vi "DDS_only.vi"() -> ()   [LabVIEW 2011]
doc: "I Description:\nThis example uses a script to manage the generation of a dynamic pattern at a specified clock rate.\n\nII Instructions for Running:\n1. Enter the digital channels on the hardware device to generate digital pattern in the Channel List control.\n2. Specify the clock rate for the generation in the Clock Rate control.\n3. Click the Stop button when you want to stop the generation\n\nIII Block Diagram Steps:\n1. Initialize for a generation session.\n2. Assign specified channels in Channel List for dynamic operation.\n3. Configure the Sample clock to use the onboard clock, and configure the clock rate.\n4. Set the generation mode to Scripted.\n5. Query the Data Width property to determine which Write function to use.\nNote: Different devices have different default values for the Data Width property. If you know the Data Width of your device, you may omit the property node and case structure.\n6. Write digital patterns to the onboard memory of the digital device.\n7. Write the script to the onboard memory.\n8. Initiate dynamic pattern generation.\n9. Wait until the Stop button is clicked or an error occurs, and exit the While loop. \n The niHSDIO Is Done VI is used in the while loop to check only for errors.\n10. Abort generation and close the session.\n\nIV I/O Connections Overview:\nMake connections from output terminals to match the channels specified by Channel List. In this example, the digital pattern is generated from the first 16 digital channels of the device."
uses:
  DDS drivers v3/DDS Settings.ctl
  DDS drivers v3/DDS RAM mode.ctl
  DDS drivers v3/DDS box device reference.ctl
  <vilib>/ni845x/ni845x.llb/ni845xControl.ctl
  ExperimentVariables/Variable_Settings.ctl
  <vilib>/Utility/error.llb/DialogType.ctl
  DDS drivers v3/AD9910 registers.ctl
  <vilib>/Utility/file.llb/Read From Spreadsheet File (string).vi
  ExperimentVariables/ExperimentVariables.lvclass
  DDS/DDS.lvclass
panel:
  in  "Quit Program":bool
  in  "Tab Control":enum32{"Experiment Variables", "DDS"}(tab)=enum."DDS"
  in  "Log":string="2012-07-23 09:53:31 Experiment ended\n\n2012-07-23 09:53:08 Experiment started\n\n2012-07-23 09:53:05 Experiment ended\n\n2012-07-23 09:52:53 Experiment started\n\n2012-07-23 09:52:48 Experiment ended\n\n2012-07-23 09:52:26 Experiment started\n\n2012-07-23 09:51:43 Experiment ended\n\n2012-07-23 09:46:17 Experiment started\n\n2012-07-23 09:44:29 Experiment ended\n\n2012-07-23 09:40:15 Experiment started\n\n2012-07-23 09:37:09 Experiment ended\n\n2012-07-23 09:32:48 Experiment started\n\n2012-07-23 09:32:41 Experiment ended\n\n2012-07-23 09:29:43 Experiment started\n\n2012-07-23 09:29:27 Experiment ended\n\n2012-07-23 09:26:51 Experiment started\n\n2012-07-23 09:26:22 Experiment ended\n\n2012-07-23 09:26:09 Experiment started\n\n2012-07-23 09:26:03 Experiment ended\n\n2012-07-23 09:25:53 Experiment started\n\n2012-07-23 09:25:46 Experiment ended\n\n2012-07-23 09:25:36 Experiment started\n\n2012-07-23 09:25:22 Experiment ended\n\n2012-07-23 09:25:08 Experiment started\n\n2012-07-23 09:24:58 Experiment ended\n\n2012-07-23 09:24:45 Experiment started\n\n2012-07-20 17:55:37 \n\nError cleared and continued by user\n\n2012-07-20 17:55:35 Warning 200010 occurred at DAQmx Stop Task.vi:4\r\n\r\nPossible reason(s):\n\r\nFinite acquisition or generation has been stopped before the requested number of samples were acquired or generated.\n\n2012-07-20 17:55:35 Experiment ended\n\n2012-07-20 17:54:26 Experiment started\n\n2012-07-20 17:53:50 Experiment ended\n\n2012-07-20 17:48:30 Experiment started\n\n2012-07-20 17:48:24 Experiment ended\n\n2012-07-20 17:43:48 Experiment started\n\n2012-07-20 17:43:47 Experiment ended\n\n2012-07-20 17:38:30 Experiment started\n\n2012-07-20 17:27:08 Experiment ended\n\n2012-07-20 17:26:09 Experiment started\n\n2012-07-20 17:25:58 \n\nError cleared and continued by user\n\n2012-07-20 17:25:57 Warning 200010 occurred at DAQmx Stop Task.vi:4\r\n\r\nPossible reason(s):\n\r\nFinite acquisition or generation has been stopped before the requested number of samples were acquired or generated.\n\n2012-07-20 17:25:57 Experiment ended\n\n2012-07-20 17:24:56 Experiment started\n\n2012-07-20 17:24:55 Experiment ended\n\n2012-07-20 17:19:07 Experiment started\n\n2012-07-20 16:57:52 Experiment ended\n\n2012-07-20 16:57:48 Experiment started\n\n2012-07-20 16:31:13 Experiment ended\n\n2012-07-20 16:28:51 Experiment started\n\n2012-07-20 16:26:58 \n\nError cleared and continued by user\n\n2012-07-20 16:26:56 Warning 200010 occurred at DAQmx Stop Task.vi:4\r\n\r\nPossible reason(s):\n\r\nFinite acquisition or generation has been stopped before the requested number of samples were acquired or generated.\n\n2012-07-20 16:26:56 Experiment ended\n\n2012-07-20 16:25:46 Experiment started\n\n2012-07-20 16:25:13 Experiment ended\n\n2012-07-20 16:25:06 Experiment started\n\n2012-07-20 16:20:49 Experiment ended\n\n2012-07-20 16:20:45 Warning:  The measurement ended due to the master timeout, before all output tasks were complete.  Consider increasing the timeout.\n\n2012-07-20 16:20:42 Warning:  The measurement ended due to the master timeout, before all output tasks were complete.  Consider increasing the timeout.\n\n2012-07-20 16:20:36 Warning:  The measurement ended due to the master timeout, before all output tasks were complete.  Consider increasing the timeout.\n\n2012-07-20 16:20:33 Warning:  The measurement ended due to the master timeout, before all output tasks were complete.  Consider increasing the timeout.\n\n2012-07-20 16:20:30 Warning:  The measurement ended due to the master timeout, before all output tasks were complete.  Consider increasing the timeout.\n\n2012-07-20 16:20:27 Warning:  The measurement ended due to the master timeout, before all output tasks were complete.  Consider increasing the timeout.\n\n2012-07-20 16:20:24 Warning:  The measurement ended due to the master timeout, before all output tasks were complete.  Consider increasing the timeout.\n\n2012-07-20 16:20:21 Warning:  The measurement ended due to the master timeout, before all output tasks were complete.  Consider increasing the timeout.\n\n2012-07-20 16:20:17 Warning:  The measurement ended due to the master timeout, before all output tasks were complete.  Consider increasing the timeout.\n\n2012-07-20 16:20:14 Warning:  The measurement ended due to the master timeout, before all output tasks were complete.  Consider increasing the timeout.\n\n2012-07-20 16:20:11 Warning:  The measurement ended due to the master timeout, before all output tasks were complete.  Consider increasing the timeout.\n\n2012-07-20 16:20:08 Warning:  The measurement ended due to the master timeout, before all output tasks were complete.  Consider increasing the timeout.\n\n2012-07-20 16:20:05 Warning:  The measurement ended due to the master timeout, before all output tasks were complete.  Consider increasing the timeout.\n\n2012-07-20 16:20:02 Warning:  The measurement ended due to the master timeout, before all output tasks were complete.  Consider increasing the timeout.\n\n2012-07-20 16:19:59 Warning:  The measurement ended due to the master timeout, before all output tasks were complete.  Consider increasing the timeout.\n\n2012-07-20 16:19:56 Warning:  The measurement ended due to the master timeout, before all output tasks were complete.  Consider increasing the timeout.\n\n2012-07-20 16:19:53 Warning:  The measurement ended due to the master timeout, before all output tasks were complete.  Consider increasing the timeout.\n\n2012-07-20 16:19:50 Warning:  The measurement ended due to the master timeout, before all output tasks were complete.  Consider increasing the timeout.\n\n2012-07-20 16:19:47 Warning:  The measurement ended due to the master timeout, before all output tasks were complete.  Consider increasing the timeout.\n\n2012-07-20 16:19:43 Warning:  The measurement ended due to the master timeout, before all output tasks were complete.  Consider increasing the timeout.\n\n2012-07-20 16:19:40 Warning:  The measurement ended due to the master timeout, before all output tasks were complete.  Consider increasing the timeout.\n\n2012-07-20 16:19:37 Warning:  The measurement ended due to the master timeout, before all output tasks were complete.  Consider increasing the timeout.\n\n2012-07-20 16:19:34 Warning:  The measurement ended due to the master timeout, before all output tasks were complete.  Consider increasing the timeout.\n\n2012-07-20 16:19:31 Warning:  The measurement ended due to the master timeout, before all output tasks were complete.  Consider increasing the timeout.\n\n2012-07-20 16:19:28 Warning:  The measurement ended due to the master timeout, before all output tasks were complete.  Consider increasing the timeout.\n\n2012-07-20 16:19:25 Warning:  The measurement ended due to the master timeout, before all output tasks were complete.  Consider increasing the timeout.\n\n2012-07-20 16:19:22 Warning:  The measurement ended due to the master timeout, before all output tasks were complete.  Consider increasing the timeout.\n\n2012-07-20 16:19:19 Warning:  The measurement ended due to the master timeout, before all output tasks were complete.  Consider increasing the timeout.\n\n2012-07-20 16:19:16 Experiment started\n\n2012-07-20 16:16:53 Experiment ended\n\n2012-07-20 16:16:51 Warning:  The measurement ended due to the master timeout, before all output tasks were complete.  Consider increasing the timeout.\n\n2012-07-20 16:16:48 Warning:  The measurement ended due to the master timeout, before all output tasks were complete.  Consider increasing the timeout.\n\n2012-07-20 16:16:45 Warning:  The measurement ended due to the master timeout, before all output tasks were complete.  Consider increasing the timeout.\n\n2012-07-20 16:16:42 Warning:  The measurement ended due to the master timeout, before all output tasks were complete.  Consider increasing the timeout.\n\n2012-07-20 16:16:39 Warning:  The measurement ended due to the master timeout, before all output tasks were complete.  Consider increasing the timeout.\n\n2012-07-20 16:16:36 Warning:  The measurement ended due to the master timeout, before all output tasks were complete.  Consider increasing the timeout.\n\n2012-07-20 16:16:33 Warning:  The measurement ended due to the master timeout, before all output tasks were complete.  Consider increasing the timeout.\n\n2012-07-20 16:16:29 Experiment started\n\n2012-07-20 16:15:09 Experiment ended\n\n2012-07-20 16:13:39 Warning:  The measurement ended due to the master timeout, before all output tasks were complete.  Consider increasing the timeout.\n\n2012-07-20 16:13:36 Warning:  The measurement ended due to the master timeout, before all output tasks were complete.  Consider increasing the timeout.\n\n2012-07-20 16:13:33 Warning:  The measurement ended due to the master timeout, before all output tasks were complete.  Consider increasing the timeout.\n\n2012-07-20 16:13:30 Warning:  The measurement ended due to the master timeout, before all output tasks were complete.  Consider increasing the timeout.\n\n2012-07-20 16:13:27 Warning:  The measurement ended due to the master timeout, before all output tasks were complete.  Consider increasing the timeout.\n\n2012-07-20 16:13:24 Warning:  The measurement ended due to the master timeout, before all output tasks were complete.  Consider increasing the timeout.\n\n2012-07-20 16:13:21 Warning:  The measurement ended due to the master timeout, before all output tasks were complete.  Consider increasing the timeout.\n\n2012-07-20 16:13:18 Warning:  The measurement ended due to the master timeout, before all output tasks were complete.  Consider increasing the timeout.\n\n2012-07-20 16:13:15 Warning:  The measurement ended due to the master timeout, before all output tasks were complete.  Consider increasing the timeout.\n\n2012-07-20 16:13:12 Warning:  The measurement ended due to the master timeout, before all output tasks were complete.  Consider increasing the timeout.\n\n2012-07-20 16:13:08 Warning:  The measurement ended due to the master timeout, before all output tasks were complete.  Consider increasing the timeout.\n\n2012-07-20 16:13:05 Warning:  The measurement ended due to the master timeout, before all output tasks were complete.  Consider increasing the timeout.\n\n2012-07-20 16:13:02 Warning:  The measurement ended due to the master timeout, before all output tasks were complete.  Consider increasing the timeout.\n\n2012-07-20 16:12:59 Warning:  The measurement ended due to the master timeout, before all output tasks were complete.  Consider increasing the timeout.\n\n2012-07-20 16:12:56 Warning:  The measurement ended due to the master timeout, before all output tasks were complete.  Consider increasing the timeout.\n\n2012-07-20 16:12:53 Warning:  The measurement ended due to the master timeout, before all output tasks were complete.  Consider increasing the timeout.\n\n2012-07-20 16:12:50 Warning:  The measurement ended due to the master timeout, before all output tasks were complete.  Consider increasing the timeout.\n\n2012-07-20 16:12:47 Warning:  The measurement ended due to the master timeout, before all output tasks were complete.  Consider increasing the timeout.\n\n2012-07-20 16:12:44 Warning:  The measurement ended due to the master timeout, before all output tasks were complete.  Consider increasing the timeout.\n\n2012-07-20 16:12:41 Warning:  The measurement ended due to the master timeout, before all output tasks were complete.  Consider increasing the timeout.\n\n2012-07-20 16:12:37 Warning:  The measurement ended due to the master timeout, before all output tasks were complete.  Consider increasing the timeout.\n\n2012-07-20 16:12:34 Warning:  The measurement ended due to the master timeout, before all output tasks were complete.  Consider increasing the timeout.\n\n2012-07-20 16:12:31 Warning:  The measurement ended due to the master timeout, before all output tasks were complete.  Consider increasing the timeout.\n\n2012-07-20 16:12:28 Warning:  The measurement ended due to the master timeout, before all output tasks were complete.  Consider increasing the timeout.\n\n2012-07-20 16:12:25 Warning:  The measurement ended due to the master timeout, before all output tasks were complete.  Consider increasing the timeout.\n\n2012-07-20 16:12:22 Warning:  The measurement ended due to the master timeout, before all output tasks were complete.  Consider increasing the timeout.\n\n2012-07-20 16:12:19 Warning:  The measurement ended due to the master timeout, before all output tasks were complete.  Consider increasing the timeout.\n\n2012-07-20 16:12:16 Warning:  The measurement ended due to the master timeout, before all output tasks were complete.  Consider increasing the timeout.\n\n2012-07-20 16:12:13 Warning:  The measurement ended due to the master timeout, before all output tasks were complete.  Consider increasing the timeout.\n\n2012-07-20 16:12:10 Warning:  The measurement ended due to the master timeout, before all output tasks were complete.  Consider increasing the timeout.\n\n2012-07-20 16:12:06 Warning:  The measurement ended due to the master timeout, before all output tasks were complete.  Consider increasing the timeout.\n\n2012-07-20 16:12:03 Warning:  The measurement ended due to the master timeout, before all output tasks were complete.  Consider increasing the timeout.\n\n2012-07-20 16:12:00 Warning:  The measurement ended due to the master timeout, before all output tasks were complete.  Consider increasing the timeout.\n\n2012-07-20 16:11:57 Warning:  The measurement ended due to the master timeout, before all output tasks were complete.  Consider increasing the timeout.\n\n2012-07-20 16:11:54 Warning:  The measurement ended due to the master timeout, before all output tasks were complete.  Consider increasing the timeout.\n\n2012-07-20 16:11:51 Warning:  The measurement ended due to the master timeout, before all output tasks were complete.  Consider increasing the timeout.\n\n2012-07-20 16:11:48 Warning:  The measurement ended due to the master timeout, before all output tasks were complete.  Consider increasing the timeout.\n\n2012-07-20 16:11:45 Warning:  The measurement ended due to the master timeout, before all output tasks were complete.  Consider increasing the timeout.\n\n2012-07-20 16:11:42 Warning:  The measurement ended due to the master timeout, before all output tasks were complete.  Consider increasing the timeout.\n\n2012-07-20 16:11:39 Warning:  The measurement ended due to the master timeout, before all output tasks were complete.  Consider increasing the timeout.\n\n2012-07-20 16:11:36 Warning:  The measurement ended due to the master timeout, before all output tasks were complete.  Consider increasing the timeout.\n\n2012-07-20 16:11:33 Warning:  The measurement ended due to the master timeout, before all output tasks were complete.  Consider increasing the timeout.\n\n2012-07-20 16:11:30 Warning:  The measurement ended due to the master timeout, before all output tasks were complete.  Consider increasing the timeout.\n\n2012-07-20 16:11:27 Warning:  The measurement ended due to the master timeout, before all output tasks were complete.  Consider increasing the timeout.\n\n2012-07-20 16:11:24 Warning:  The measurement ended due to the master timeout, before all output tasks were complete.  Consider increasing the timeout.\n\n2012-07-20 16:11:21 Warning:  The measurement ended due to the master timeout, before all output tasks were complete.  Consider increasing the timeout.\n\n2012-07-20 16:11:18 Warning:  The measurement ended due to the master timeout, before all output tasks were complete.  Consider increasing the timeout.\n\n2012-07-20 16:11:15 Warning:  The measurement ended due to the master timeout, before all output tasks were complete.  Consider increasing the timeout.\n\n2012-07-20 16:11:12 Warning:  The measurement ended due to the master timeout, before all output tasks were complete.  Consider increasing the timeout.\n\n2012-07-20 16:11:09 Warning:  The measurement ended due to the master timeout, before all output tasks were complete.  Consider increasing the timeout.\n\n2012-07-20 16:11:05 Warning:  The measurement ended due to the master timeout, before all output tasks were complete.  Consider increasing the timeout.\n\n2012-07-20 16:11:02 Warning:  The measurement ended due to the master timeout, before all output tasks were complete.  Consider increasing the timeout.\n\n2012-07-20 16:10:59 Warning:  The measurement ended due to the master timeout, before all output tasks were complete.  Consider increasing the timeout.\n\n2012-07-20 16:10:56 Warning:  The measurement ended due to the master timeout, before all output tasks were complete.  Consider increasing the timeout.\n\n2012-07-20 16:10:53 Warning:  The measurement ended due to the master timeout, before all output tasks were complete.  Consider increasing the timeout.\n\n2012-07-20 16:10:50 Warning:  The measurement ended due to the master timeout, before all output tasks were complete.  Consider increasing the timeout.\n\n2012-07-20 16:10:47 Warning:  The measurement ended due to the master timeout, before all output tasks were complete.  Consider increasing the timeout.\n\n2012-07-20 16:10:44 Warning:  The measurement ended due to the master timeout, before all output tasks were complete.  Consider increasing the timeout.\n\n2012-07-20 16:10:41 Warning:  The measurement ended due to the master timeout, before all output tasks were complete.  Consider increasing the timeout.\n\n2012-07-20 16:10:38 Warning:  The measurement ended due to the master timeout, before all output tasks were complete.  Consider increasing the timeout.\n\n2012-07-20 16:10:34 Warning:  The measurement ended due to the master timeout, before all output tasks were complete.  Consider increasing the timeout.\n\n2012-07-20 16:10:31 Warning:  The measurement ended due to the master timeout, before all output tasks were complete.  Consider increasing the timeout.\n\n2012-07-20 16:10:28 Warning:  The measurement ended due to the master timeout, before all output tasks were complete.  Consider increasing the timeout.\n\n2012-07-20 16:10:25 Warning:  The measurement ended due to the master timeout, before all output tasks were complete.  Consider increasing the timeout.\n\n2012-07-20 16:10:22 Warning:  The measurement ended due to the master timeout, before all output tasks were complete.  Consider increasing the timeout.\n\n2012-07-20 16:10:19 Warning:  The measurement ended due to the master timeout, before all output tasks were complete.  Consider increasing the timeout.\n\n2012-07-20 16:10:16 Warning:  The measurement ended due to the master timeout, before all output tasks were complete.  Consider increasing the timeout.\n\n2012-07-20 16:10:13 Warning:  The measurement ended due to the master timeout, before all output tasks were complete.  Consider increasing the timeout.\n\n2012-07-20 16:10:10 Warning:  The measurement ended due to the master timeout, before all output tasks were complete.  Consider increasing the timeout.\n\n2012-07-20 16:10:07 Warning:  The measurement ended due to the master timeout, before all output tasks were complete.  Consider increasing the timeout.\n\n2012-07-20 16:10:03 Warning:  The measurement ended due to the master timeout, before all output tasks were complete.  Consider increasing the timeout.\n\n2012-07-20 16:10:00 Warning:  The measurement ended due to the master timeout, before all output tasks were complete.  Consider increasing the timeout.\n\n2012-07-20 16:09:57 Warning:  The measurement ended due to the master timeout, before all output tasks were complete.  Consider increasing the timeout.\n\n2012-07-20 16:09:54 Warning:  The measurement ended due to the master timeout, before all output tasks were complete.  Consider increasing the timeout.\n\n2012-07-20 16:09:51 Warning:  The measurement ended due to the master timeout, before all output tasks were complete.  Consider increasing the timeout.\n\n2012-07-20 16:09:48 Warning:  The measurement ended due to the master timeout, before all output tasks were complete.  Consider increasing the timeout.\n\n2012-07-20 16:09:45 Warning:  The measurement ended due to the master timeout, before all output tasks were complete.  Consider increasing the timeout.\n\n2012-07-20 16:09:42 Warning:  The measurement ended due to the master timeout, before all output tasks were complete.  Consider increasing the timeout.\n\n2012-07-20 16:09:39 Warning:  The measurement ended due to the master timeout, before all output tasks were complete.  Consider increasing the timeout.\n\n2012-07-20 16:09:36 Warning:  The measurement ended due to the master timeout, before all output tasks were complete.  Consider increasing the timeout.\n\n2012-07-20 16:09:33 Warning:  The measurement ended due to the master timeout, before all output tasks were complete.  Consider increasing the timeout.\n\n2012-07-20 16:09:30 Warning:  The measurement ended due to the master timeout, before all output tasks were complete.  Consider increasing the timeout.\n\n2012-07-20 16:09:27 Warning:  The measurement ended due to the master timeout, before all output tasks were complete.  Consider increasing the timeout.\n\n2012-07-20 16:09:24 Warning:  The measurement ended due to the master timeout, before all output tasks were complete.  Consider increasing the timeout.\n\n2012-07-20 16:09:21 Warning:  The measurement ended due to the master timeout, before all output tasks were complete.  Consider increasing the timeout.\n\n2012-07-20 16:09:18 Warning:  The measurement ended due to the master timeout, before all output tasks were complete.  Consider increasing the timeout.\n\n2012-07-20 16:09:15 Warning:  The measurement ended due to the master timeout, before all output tasks were complete.  Consider increasing the timeout.\n\n2012-07-20 16:09:12 Warning:  The measurement ended due to the master timeout, before all output tasks were complete.  Consider increasing the timeout.\n\n2012-07-20 16:09:09 Warning:  The measurement ended due to the master timeout, before all output tasks were complete.  Consider increasing the timeout.\n\n2012-07-20 16:09:06 Warning:  The measurement ended due to the master timeout, before all output tasks were complete.  Consider increasing the timeout.\n\n2012-07-20 16:09:02 Warning:  The measurement ended due to the master timeout, before all output tasks were complete.  Consider increasing the timeout.\n\n2012-07-20 16:08:59 Warning:  The measurement ended due to the master timeout, before all output tasks were complete.  Consider increasing the timeout.\n\n2012-07-20 16:08:56 Warning:  The measurement ended due to the master timeout, before all output tasks were complete.  Consider increasing the timeout.\n\n2012-07-20 16:08:53 Warning:  The measurement ended due to the master timeout, before all output tasks were complete.  Consider increasing the timeout.\n\n2012-07-20 16:08:50 Warning:  The measurement ended due to the master timeout, before all output tasks were complete.  Consider increasing the timeout.\n\n2012-07-20 16:08:47 Warning:  The measurement ended due to the master timeout, before all output tasks were complete.  Consider increasing the timeout.\n\n2012-07-20 16:08:44 Warning:  The measurement ended due to the master timeout, before all output tasks were complete.  Consider increasing the timeout.\n\n2012-07-20 16:08:38 Warning:  The measurement ended due to the master timeout, before all output tasks were complete.  Consider increasing the timeout.\n\n2012-07-20 16:08:35 Warning:  The measurement ended due to the master timeout, before all output tasks were complete.  Consider increasing the timeout.\n\n2012-07-20 16:08:31 Warning:  The measurement ended due to the master timeout, before all output tasks were complete.  Consider increasing the timeout.\n\n2012-07-20 16:08:28 Warning:  The measurement ended due to the master timeout, before all output tasks were complete.  Consider increasing the timeout.\n\n2012-07-20 16:08:25 Warning:  The measurement ended due to the master timeout, before all output tasks were complete.  Consider increasing the timeout.\n\n2012-07-20 16:08:22 Warning:  The measurement ended due to the master timeout, before all output tasks were complete.  Consider increasing the timeout.\n\n2012-07-20 16:08:19 Warning:  The measurement ended due to the master timeout, before all output tasks were complete.  Consider increasing the timeout.\n\n2012-07-20 16:08:16 Warning:  The measurement ended due to the master timeout, before all output tasks were complete.  Consider increasing the timeout.\n\n2012-07-20 16:08:13 Warning:  The measurement ended due to the master timeout, before all output tasks were complete.  Consider increasing the timeout.\n\n2012-07-20 16:08:10 Warning:  The measurement ended due to the master timeout, before all output tasks were complete.  Consider increasing the timeout.\n\n2012-07-20 16:08:07 Warning:  The measurement ended due to the master timeout, before all output tasks were complete.  Consider increasing the timeout.\n\n2012-07-20 16:08:04 Warning:  The measurement ended due to the master timeout, before all output tasks were complete.  Consider increasing the timeout.\n\n2012-07-20 16:08:00 Experiment started\n\n2012-07-20 16:07:21 \n\nHalted by user.\n\n2012-07-20 16:07:18 Error -50103 occurred at Analog_Output.lvclass:update.vi\r\n\r\nPossible reason(s):\n\r\nNI Platform Services:  The specified resource is reserved. The operation could not be completed as specified.\r\n\nTask Name: _unnamedTask<185>\n\n2012-07-20 16:07:18 Experiment ended\n\n2012-07-20 16:07:16 Experiment started\n\n2012-07-20 16:07:16 \n\nError cleared and continued by user\n\n2012-07-20 16:07:14 Error 100 occurred at DDS Com Error\r\n\r\nPossible reason(s):\n\r\nLabVIEW:  File contains erroneous data. This normally is a user data file.\n\n2012-07-20 16:07:14 Experiment ended\n\n2012-07-20 16:07:12 Experiment started\n\n2012-07-20 16:06:57 \n\nHalted by user.\n\n2012-07-20 16:06:46 Error 100 occurred at DDS Com Error\r\n\r\nPossible reason(s):\n\r\nLabVIEW:  File contains erroneous data. This normally is a user data file.\n\n2012-07-20 16:06:46 Experiment ended\n\n2012-07-20 16:06:38 Experiment started\n\n2012-07-20 16:06:13 \n\nError cleared and continued by user\n\n2012-07-20 16:06:10 Error 100 occurred at DDS Com Error\r\n\r\nPossible reason(s):\n\r\nLabVIEW:  File contains erroneous data. This normally is a user data file.\n\n2012-07-20 16:06:10 Experiment ended\n\n2012-07-20 16:06:06 Experiment started\n\n2012-07-20 16:05:54 \n\nError cleared and continued by user\n\n2012-07-20 16:05:52 Error 100 occurred at DDS Com Error\r\n\r\nPossible reason(s):\n\r\nLabVIEW:  File contains erroneous data. This normally is a user data file.\n\n2012-07-20 16:05:52 Experiment ended\n\n2012-07-20 16:05:49 Experiment started\n\n2012-07-20 16:05:16 Experiment ended\n\n2012-07-20 16:04:44 Warning:  The measurement ended due to the master timeout, before all output tasks were complete.  Consider increasing the timeout.\n\n2012-07-20 16:04:41 Warning:  The measurement ended due to the master timeout, before all output tasks were complete.  Consider increasing the timeout.\n\n2012-07-20 16:04:38 Warning:  The measurement ended due to the master timeout, before all output tasks were complete.  Consider increasing the timeout.\n\n2012-07-20 16:04:35 Warning:  The measurement ended due to the master timeout, before all output tasks were complete.  Consider increasing the timeout.\n\n2012-07-20 16:04:31 Warning:  The measurement ended due to the master timeout, before all output tasks were complete.  Consider increasing the timeout.\n\n2012-07-20 16:04:28 Warning:  The measurement ended due to the master timeout, before all output tasks were complete.  Consider increasing the timeout.\n\n2012-07-20 16:04:25 Warning:  The measurement ended due to the master timeout, before all output tasks were complete.  Consider increasing the timeout.\n\n2012-07-20 16:04:22 Warning:  The measurement ended due to the master timeout, before all output tasks were complete.  Consider increasing the timeout.\n\n2012-07-20 16:04:19 Warning:  The measurement ended due to the master timeout, before all output tasks were complete.  Consider increasing the timeout.\n\n2012-07-20 16:04:16 Warning:  The measurement ended due to the master timeout, before all output tasks were complete.  Consider increasing the timeout.\n\n2012-07-20 16:04:13 Warning:  The measurement ended due to the master timeout, before all output tasks were complete.  Consider increasing the timeout.\n\n2012-07-20 16:04:10 Warning:  The measurement ended due to the master timeout, before all output tasks were complete.  Consider increasing the timeout.\n\n2012-07-20 16:04:07 Warning:  The measurement ended due to the master timeout, before all output tasks were complete.  Consider increasing the timeout.\n\n2012-07-20 16:04:04 Warning:  The measurement ended due to the master timeout, before all output tasks were complete.  Consider increasing the timeout.\n\n2012-07-20 16:04:01 Warning:  The measurement ended due to the master timeout, before all output tasks were complete.  Consider increasing the timeout.\n\n2012-07-20 16:03:58 Warning:  The measurement ended due to the master timeout, before all output tasks were complete.  Consider increasing the timeout.\n\n2012-07-20 16:03:55 Warning:  The measurement ended due to the master timeout, before all output tasks were complete.  Consider increasing the timeout.\n\n2012-07-20 16:03:51 Warning:  The measurement ended due to the master timeout, before all output tasks were complete.  Consider increasing the timeout.\n\n2012-07-20 16:03:48 Warning:  The measurement ended due to the master timeout, before all output tasks were complete.  Consider increasing the timeout.\n\n2012-07-20 16:03:45 Warning:  The measurement ended due to the master timeout, before all output tasks were complete.  Consider increasing the timeout.\n\n2012-07-20 16:03:42 Warning:  The measurement ended due to the master timeout, before all output tasks were complete.  Consider increasing the timeout.\n\n2012-07-20 16:03:39 Warning:  The measurement ended due to the master timeout, before all output tasks were complete.  Consider increasing the timeout.\n\n2012-07-20 16:03:36 Warning:  The measurement ended due to the master timeout, before all output tasks were complete.  Consider increasing the timeout.\n\n2012-07-20 16:03:33 Warning:  The measurement ended due to the master timeout, before all output tasks were complete.  Consider increasing the timeout.\n\n2012-07-20 16:03:30 Warning:  The measurement ended due to the master timeout, before all output tasks were complete.  Consider increasing the timeout.\n\n2012-07-20 16:03:27 Warning:  The measurement ended due to the master timeout, before all output tasks were complete.  Consider increasing the timeout.\n\n2012-07-20 16:03:24 Warning:  The measurement ended due to the master timeout, before all output tasks were complete.  Consider increasing the timeout.\n\n2012-07-20 16:03:21 Warning:  The measurement ended due to the master timeout, before all output tasks were complete.  Consider increasing the timeout.\n\n2012-07-20 16:03:18 Warning:  The measurement ended due to the master timeout, before all output tasks were complete.  Consider increasing the timeout.\n\n2012-07-20 16:03:15 Warning:  The measurement ended due to the master timeout, before all output tasks were complete.  Consider increasing the timeout.\n\n2012-07-20 16:03:12 Warning:  The measurement ended due to the master timeout, before all output tasks were complete.  Consider increasing the timeout.\n\n2012-07-20 16:03:09 Warning:  The measurement ended due to the master timeout, before all output tasks were complete.  Consider increasing the timeout.\n\n2012-07-20 16:03:05 Warning:  The measurement ended due to the master timeout, before all output tasks were complete.  Consider increasing the timeout.\n\n2012-07-20 16:03:02 Warning:  The measurement ended due to the master timeout, before all output tasks were complete.  Consider increasing the timeout.\n\n2012-07-20 16:02:59 Warning:  The measurement ended due to the master timeout, before all output tasks were complete.  Consider increasing the timeout.\n\n2012-07-20 16:02:56 Warning:  The measurement ended due to the master timeout, before all output tasks were complete.  Consider increasing the timeout.\n\n2012-07-20 16:02:53 Warning:  The measurement ended due to the master timeout, before all output tasks were complete.  Consider increasing the timeout.\n\n2012-07-20 16:02:50 Warning:  The measurement ended due to the master timeout, before all output tasks were complete.  Consider increasing the timeout.\n\n2012-07-20 16:02:47 Warning:  The measurement ended due to the master timeout, before all output tasks were complete.  Consider increasing the timeout.\n\n2012-07-20 16:02:44 Warning:  The measurement ended due to the master timeout, before all output tasks were complete.  Consider increasing the timeout.\n\n2012-07-20 16:02:41 Warning:  The measurement ended due to the master timeout, before all output tasks were complete.  Consider increasing the timeout.\n\n2012-07-20 16:02:38 Warning:  The measurement ended due to the master timeout, before all output tasks were complete.  Consider increasing the timeout.\n\n2012-07-20 16:02:35 Warning:  The measurement ended due to the master timeout, before all output tasks were complete.  Consider increasing the timeout.\n\n2012-07-20 16:02:32 Warning:  The measurement ended due to the master timeout, before all output tasks were complete.  Consider increasing the timeout.\n\n2012-07-20 16:02:28 Warning:  The measurement ended due to the master timeout, before all output tasks were complete.  Consider increasing the timeout.\n\n2012-07-20 16:02:25 Warning:  The measurement ended due to the master timeout, before all output tasks were complete.  Consider increasing the timeout.\n\n2012-07-20 16:02:19 Warning:  The measurement ended due to the master timeout, before all output tasks were complete.  Consider increasing the timeout.\n\n2012-07-20 16:02:16 Warning:  The measurement ended due to the master timeout, before all output tasks were complete.  Consider increasing the timeout.\n\n2012-07-20 16:02:13 Warning:  The measurement ended due to the master timeout, before all output tasks were complete.  Consider increasing the timeout.\n\n2012-07-20 16:02:10 Warning:  The measurement ended due to the master timeout, before all output tasks were complete.  Consider increasing the timeout.\n\n2012-07-20 16:02:07 Warning:  The measurement ended due to the master timeout, before all output tasks were complete.  Consider increasing the timeout.\n\n2012-07-20 16:02:04 Warning:  The measurement ended due to the master timeout, before all output tasks were complete.  Consider increasing the timeout.\n\n2012-07-20 16:02:01 Warning:  The measurement ended due to the master timeout, before all output tasks were complete.  Consider increasing the timeout.\n\n2012-07-20 16:01:57 Warning:  The measurement ended due to the master timeout, before all output tasks were complete.  Consider increasing the timeout.\n\n2012-07-20 16:01:54 Warning:  The measurement ended due to the master timeout, before all output tasks were complete.  Consider increasing the timeout.\n\n2012-07-20 16:01:51 Warning:  The measurement ended due to the master timeout, before all output tasks were complete.  Consider increasing the timeout.\n\n2012-07-20 16:01:48 Warning:  The measurement ended due to the master timeout, before all output tasks were complete.  Consider increasing the timeout.\n\n2012-07-20 16:01:45 Warning:  The measurement ended due to the master timeout, before all output tasks were complete.  Consider increasing the timeout.\n\n2012-07-20 16:01:42 Warning:  The measurement ended due to the master timeout, before all output tasks were complete.  Consider increasing the timeout.\n\n2012-07-20 16:01:39 Warning:  The measurement ended due to the master timeout, before all output tasks were complete.  Consider increasing the timeout.\n\n2012-07-20 16:01:36 Warning:  The measurement ended due to the master timeout, before all output tasks were complete.  Consider increasing the timeout.\n\n2012-07-20 16:01:33 Warning:  The measurement ended due to the master timeout, before all output tasks were complete.  Consider increasing the timeout.\n\n2012-07-20 16:01:30 Warning:  The measurement ended due to the master timeout, before all output tasks were complete.  Consider increasing the timeout.\n\n2012-07-20 16:01:23 Warning:  The measurement ended due to the master timeout, before all output tasks were complete.  Consider increasing the timeout.\n\n2012-07-20 16:01:20 Warning:  The measurement ended due to the master timeout, before all output tasks were complete.  Consider increasing the timeout.\n\n2012-07-20 16:01:17 Warning:  The measurement ended due to the master timeout, before all output tasks were complete.  Consider increasing the timeout.\n\n2012-07-20 16:01:14 Warning:  The measurement ended due to the master timeout, before all output tasks were complete.  Consider increasing the timeout.\n\n2012-07-20 16:01:11 Warning:  The measurement ended due to the master timeout, before all output tasks were complete.  Consider increasing the timeout.\n\n2012-07-20 16:01:08 Warning:  The measurement ended due to the master timeout, before all output tasks were complete.  Consider increasing the timeout.\n\n2012-07-20 16:01:05 Warning:  The measurement ended due to the master timeout, before all output tasks were complete.  Consider increasing the timeout.\n\n2012-07-20 16:01:02 Warning:  The measurement ended due to the master timeout, before all output tasks were complete.  Consider increasing the timeout.\n\n2012-07-20 16:00:59 Warning:  The measurement ended due to the master timeout, before all output tasks were complete.  Consider increasing the timeout.\n\n2012-07-20 16:00:55 Warning:  The measurement ended due to the master timeout, before all output tasks were complete.  Consider increasing the timeout.\n\n2012-07-20 16:00:52 Warning:  The measurement ended due to the master timeout, before all output tasks were complete.  Consider increasing the timeout.\n\n2012-07-20 16:00:49 Warning:  The measurement ended due to the master timeout, before all output tasks were complete.  Consider increasing the timeout.\n\n2012-07-20 16:00:46 Warning:  The measurement ended due to the master timeout, before all output tasks were complete.  Consider increasing the timeout.\n\n2012-07-20 16:00:43 Warning:  The measurement ended due to the master timeout, before all output tasks were complete.  Consider increasing the timeout.\n\n2012-07-20 16:00:40 Warning:  The measurement ended due to the master timeout, before all output tasks were complete.  Consider increasing the timeout.\n\n2012-07-20 16:00:37 Warning:  The measurement ended due to the master timeout, before all output tasks were complete.  Consider increasing the timeout.\n\n2012-07-20 16:00:34 Warning:  The measurement ended due to the master timeout, before all output tasks were complete.  Consider increasing the timeout.\n\n2012-07-20 16:00:31 Warning:  The measurement ended due to the master timeout, before all output tasks were complete.  Consider increasing the timeout.\n\n2012-07-20 16:00:28 Warning:  The measurement ended due to the master timeout, before all output tasks were complete.  Consider increasing the timeout.\n\n2012-07-20 16:00:25 Warning:  The measurement ended due to the master timeout, before all output tasks were complete.  Consider increasing the timeout.\n\n2012-07-20 16:00:21 Warning:  The measurement ended due to the master timeout, before all output tasks were complete.  Consider increasing the timeout.\n\n2012-07-20 16:00:18 Warning:  The measurement ended due to the master timeout, before all output tasks were complete.  Consider increasing the timeout.\n\n2012-07-20 16:00:15 Warning:  The measurement ended due to the master timeout, before all output tasks were complete.  Consider increasing the timeout.\n\n2012-07-20 16:00:12 Warning:  The measurement ended due to the master timeout, before all output tasks were complete.  Consider increasing the timeout.\n\n2012-07-20 16:00:09 Warning:  The measurement ended due to the master timeout, before all output tasks were complete.  Consider increasing the timeout.\n\n2012-07-20 16:00:06 Warning:  The measurement ended due to the master timeout, before all output tasks were complete.  Consider increasing the timeout.\n\n2012-07-20 16:00:03 Warning:  The measurement ended due to the master timeout, before all output tasks were complete.  Consider increasing the timeout.\n\n2012-07-20 16:00:00 Warning:  The measurement ended due to the master timeout, before all output tasks were complete.  Consider increasing the timeout.\n\n2012-07-20 15:59:57 Warning:  The measurement ended due to the master timeout, before all output tasks were complete.  Consider increasing the timeout.\n\n2012-07-20 15:59:54 Experiment started\n\n2012-07-20 15:59:36 \n\nError cleared and continued by user\n\n2012-07-20 15:59:35 Warning 200010 occurred at DAQmx Stop Task.vi:4\r\n\r\nPossible reason(s):\n\r\nFinite acquisition or generation has been stopped before the requested number of samples were acquired or generated.\n\n2012-07-20 15:59:35 Experiment ended\n\n2012-07-20 15:57:39 Experiment started\n\n2012-07-20 15:52:08 \n\nError cleared and continued by user\n\n2012-07-20 15:52:06 Warning 200010 occurred at DAQmx Stop Task.vi:4\r\n\r\nPossible reason(s):\n\r\nFinite acquisition or generation has been stopped before the requested number of samples were acquired or generated.\n\n2012-07-20 15:52:06 Experiment ended\n\n2012-07-20 15:52:03 Warning:  The measurement ended due to the master timeout, before all output tasks were complete.  Consider increasing the timeout.\n\n2012-07-20 15:52:00 Warning:  The measurement ended due to the master timeout, before all output tasks were complete.  Consider increasing the timeout.\n\n2012-07-20 15:51:57 Warning:  The measurement ended due to the master timeout, before all output tasks were complete.  Consider increasing the timeout.\n\n2012-07-20 15:51:54 Warning:  The measurement ended due to the master timeout, before all output tasks were complete.  Consider increasing the timeout.\n\n2012-07-20 15:51:51 Warning:  The measurement ended due to the master timeout, before all output tasks were complete.  Consider increasing the timeout.\n\n2012-07-20 15:51:48 Warning:  The measurement ended due to the master timeout, before all output tasks were complete.  Consider increasing the timeout.\n\n2012-07-20 15:51:45 Warning:  The measurement ended due to the master timeout, before all output tasks were complete.  Consider increasing the timeout.\n\n2012-07-20 15:51:42 Warning:  The measurement ended due to the master timeout, before all output tasks were complete.  Consider increasing the timeout.\n\n2012-07-20 15:51:39 Warning:  The measurement ended due to the master timeout, before all output tasks were complete.  Consider increasing the timeout.\n\n2012-07-20 15:51:36 Warning:  The measurement ended due to the master timeout, before all output tasks were complete.  Consider increasing the timeout.\n\n2012-07-20 15:51:33 Warning:  The measurement ended due to the master timeout, before all output tasks were complete.  Consider increasing the timeout.\n\n2012-07-20 15:51:30 Warning:  The measurement ended due to the master timeout, before all output tasks were complete.  Consider increasing the timeout.\n\n2012-07-20 15:51:27 Warning:  The measurement ended due to the master timeout, before all output tasks were complete.  Consider increasing the timeout.\n\n2012-07-20 15:51:24 Warning:  The measurement ended due to the master timeout, before all output tasks were complete.  Consider increasing the timeout.\n\n2012-07-20 15:51:21 Warning:  The measurement ended due to the master timeout, before all output tasks were complete.  Consider increasing the timeout.\n\n2012-07-20 15:51:18 Warning:  The measurement ended due to the master timeout, before all output tasks were complete.  Consider increasing the timeout.\n\n2012-07-20 15:51:15 Warning:  The measurement ended due to the master timeout, before all output tasks were complete.  Consider increasing the timeout.\n\n2012-07-20 15:51:12 Warning:  The measurement ended due to the master timeout, before all output tasks were complete.  Consider increasing the timeout.\n\n2012-07-20 15:51:09 Warning:  The measurement ended due to the master timeout, before all output tasks were complete.  Consider increasing the timeout.\n\n2012-07-20 15:51:02 Warning:  The measurement ended due to the master timeout, before all output tasks were complete.  Consider increasing the timeout.\n\n2012-07-20 15:50:59 Warning:  The measurement ended due to the master timeout, before all output tasks were complete.  Consider increasing the timeout.\n\n2012-07-20 15:50:56 Warning:  The measurement ended due to the master timeout, before all output tasks were complete.  Consider increasing the timeout.\n\n2012-07-20 15:50:53 Warning:  The measurement ended due to the master timeout, before all output tasks were complete.  Consider increasing the timeout.\n\n2012-07-20 15:50:50 Warning:  The measurement ended due to the master timeout, before all output tasks were complete.  Consider increasing the timeout.\n\n2012-07-20 15:50:44 Warning:  The measurement ended due to the master timeout, before all output tasks were complete.  Consider increasing the timeout.\n\n2012-07-20 15:50:41 Warning:  The measurement ended due to the master timeout, before all output tasks were complete.  Consider increasing the timeout.\n\n2012-07-20 15:50:38 Warning:  The measurement ended due to the master timeout, before all output tasks were complete.  Consider increasing the timeout.\n\n2012-07-20 15:50:35 Warning:  The measurement ended due to the master timeout, before all output tasks were complete.  Consider increasing the timeout.\n\n2012-07-20 15:50:32 Warning:  The measurement ended due to the master timeout, before all output tasks were complete.  Consider increasing the timeout.\n\n2012-07-20 15:50:29 Warning:  The measurement ended due to the master timeout, before all output tasks were complete.  Consider increasing the timeout.\n\n2012-07-20 15:50:26 Warning:  The measurement ended due to the master timeout, before all output tasks were complete.  Consider increasing the timeout.\n\n2012-07-20 15:50:23 Warning:  The measurement ended due to the master timeout, before all output tasks were complete.  Consider increasing the timeout.\n\n2012-07-20 15:50:20 Warning:  The measurement ended due to the master timeout, before all output tasks were complete.  Consider increasing the timeout.\n\n2012-07-20 15:50:17 Warning:  The measurement ended due to the master timeout, before all output tasks were complete.  Consider increasing the timeout.\n\n2012-07-20 15:50:14 Warning:  The measurement ended due to the master timeout, before all output tasks were complete.  Consider increasing the timeout.\n\n2012-07-20 15:50:11 Warning:  The measurement ended due to the master timeout, before all output tasks were complete.  Consider increasing the timeout.\n\n2012-07-20 15:50:08 Warning:  The measurement ended due to the master timeout, before all output tasks were complete.  Consider increasing the timeout.\n\n2012-07-20 15:50:05 Warning:  The measurement ended due to the master timeout, before all output tasks were complete.  Consider increasing the timeout.\n\n2012-07-20 15:50:02 Warning:  The measurement ended due to the master timeout, before all output tasks were complete.  Consider increasing the timeout.\n\n2012-07-20 15:49:56 Warning:  The measurement ended due to the master timeout, before all output tasks were complete.  Consider increasing the timeout.\n\n2012-07-20 15:49:53 Warning:  The measurement ended due to the master timeout, before all output tasks were complete.  Consider increasing the timeout.\n\n2012-07-20 15:49:50 Warning:  The measurement ended due to the master timeout, before all output tasks were complete.  Consider increasing the timeout.\n\n2012-07-20 15:49:47 Warning:  The measurement ended due to the master timeout, before all output tasks were complete.  Consider increasing the timeout.\n\n2012-07-20 15:49:44 Warning:  The measurement ended due to the master timeout, before all output tasks were complete.  Consider increasing the timeout.\n\n2012-07-20 15:49:41 Warning:  The measurement ended due to the master timeout, before all output tasks were complete.  Consider increasing the timeout.\n\n2012-07-20 15:49:38 Warning:  The measurement ended due to the master timeout, before all output tasks were complete.  Consider increasing the timeout.\n\n2012-07-20 15:49:35 Warning:  The measurement ended due to the master timeout, before all output tasks were complete.  Consider increasing the timeout.\n\n2012-07-20 15:49:32 Warning:  The measurement ended due to the master timeout, before all output tasks were complete.  Consider increasing the timeout.\n\n2012-07-20 15:49:29 Warning:  The measurement ended due to the master timeout, before all output tasks were complete.  Consider increasing the timeout.\n\n2012-07-20 15:49:26 Warning:  The measurement ended due to the master timeout, before all output tasks were complete.  Consider increasing the timeout.\n\n2012-07-20 15:49:23 Warning:  The measurement ended due to the master timeout, before all output tasks were complete.  Consider increasing the timeout.\n\n2012-07-20 15:33:14 Warning:  The measurement ended due to the master timeout, before all output tasks were complete.  Consider increasing the timeout.\n\n2012-07-20 15:33:08 Warning:  The measurement ended due to the master timeout, before all output tasks were complete.  Consider increasing the timeout.\n\n2012-07-20 15:33:05 Warning:  The measurement ended due to the master timeout, before all output tasks were complete.  Consider increasing the timeout.\n\n2012-07-20 15:33:02 Warning:  The measurement ended due to the master timeout, before all output tasks were complete.  Consider increasing the timeout.\n\n2012-07-20 15:32:59 Warning:  The measurement ended due to the master timeout, before all output tasks were complete.  Consider increasing the timeout.\n\n2012-07-20 15:32:56 Warning:  The measurement ended due to the master timeout, before all output tasks were complete.  Consider increasing the timeout.\n\n2012-07-20 15:32:53 Warning:  The measurement ended due to the master timeout, before all output tasks were complete.  Consider increasing the timeout.\n\n2012-07-20 15:32:50 Warning:  The measurement ended due to the master timeout, before all output tasks were complete.  Consider increasing the timeout.\n\n2012-07-20 15:32:47 Warning:  The measurement ended due to the master timeout, before all output tasks were complete.  Consider increasing the timeout.\n\n2012-07-20 15:32:44 Warning:  The measurement ended due to the master timeout, before all output tasks were complete.  Consider increasing the timeout.\n\n2012-07-20 15:32:41 Warning:  The measurement ended due to the master timeout, before all output tasks were complete.  Consider increasing the timeout.\n\n2012-07-20 15:32:38 Warning:  The measurement ended due to the master timeout, before all output tasks were complete.  Consider increasing the timeout.\n\n2012-07-20 15:32:35 Warning:  The measurement ended due to the master timeout, before all output tasks were complete.  Consider increasing the timeout.\n\n2012-07-20 15:32:31 Experiment started\n\n2012-07-20 15:28:24 \n\nError cleared and continued by user\n\n2012-07-20 15:28:22 Warning 200010 occurred at DAQmx Stop Task.vi:4\r\n\r\nPossible reason(s):\n\r\nFinite acquisition or generation has been stopped before the requested number of samples were acquired or generated.\n\n2012-07-20 15:28:22 Experiment ended\n\n2012-07-20 15:28:15 Experiment started\n\n2012-07-20 15:27:01 Experiment ended\n\n2012-07-20 15:24:24 Experiment started\n\n2012-07-20 15:24:23 Experiment ended\n\n2012-07-20 15:19:58 Experiment started\n\n2012-07-20 15:15:52 Experiment ended\n\n2012-07-20 15:15:43 Experiment started\n\n2012-07-20 15:13:02 Experiment ended\n\n2012-07-20 15:11:35 Experiment started\n\n2012-07-20 15:09:20 \n\nError cleared and continued by user\n\n2012-07-20 15:09:19 Warning 200010 occurred at DAQmx Stop Task.vi:4\r\n\r\nPossible reason(s):\n\r\nFinite acquisition or generation has been stopped before the requested number of samples were acquired or generated.\n\n2012-07-20 15:09:19 Experiment ended\n\n2012-07-20 15:08:06 Experiment started\n\n2012-07-20 15:04:32 Experiment ended\n\n2012-07-20 15:00:18 Experiment started\n\n2012-07-20 15:00:06 Experiment ended\n\n2012-07-20 14:59:50 Experiment started\n\n2012-07-20 14:59:03 Experiment ended\n\n2012-07-20 14:57:14 Experiment started\n\n2012-07-20 14:56:53 Experiment ended\n\n2012-07-20 14:56:28 Experiment started\n\n2012-07-20 14:56:25 Experiment ended\n\n2012-07-20 14:56:14 Experiment started\n\n2012-07-20 14:56:08 Experiment ended\n\n2012-07-20 14:55:57 Experiment started\n\n2012-07-20 14:55:56 Experiment ended\n\n2012-07-20 14:55:38 Experiment started\n\n2012-07-20 14:55:35 Experiment ended\n\n2012-07-20 14:55:24 Experiment started\n\n2012-07-20 14:55:20 Experiment ended\n\n2012-07-20 14:55:10 Experiment started\n\n2012-07-20 14:55:03 Experiment ended\n\n2012-07-20 14:54:53 Experiment started\n\n2012-07-20 14:54:46 Experiment ended\n\n2012-07-20 14:54:35 Experiment started\n\n2012-07-20 14:54:33 Experiment ended\n\n2012-07-20 14:54:22 Experiment started\n\n2012-07-20 14:54:19 Experiment ended\n\n2012-07-20 14:54:09 Experiment started\n\n2012-07-20 14:54:06 Experiment ended\n\n2012-07-20 14:53:56 Experiment started\n\n2012-07-20 14:53:50 Experiment ended\n\n2012-07-20 14:53:39 Experiment started\n\n2012-07-20 14:53:34 Experiment ended\n\n2012-07-20 14:53:25 Experiment started\n\n2012-07-20 14:53:20 Experiment ended\n\n2012-07-20 14:53:10 Experiment started\n\n2012-07-20 14:53:00 Experiment ended\n\n2012-07-20 14:52:49 Experiment started\n\n2012-07-20 14:52:41 Experiment ended\n\n2012-07-20 14:52:31 Experiment started\n\n2012-07-20 14:52:27 Experiment ended\n\n2012-07-20 14:52:16 Experiment started\n\n2012-07-20 14:52:12 Experiment ended\n\n2012-07-20 14:52:00 Experiment started\n\n2012-07-20 14:51:56 Experiment ended\n\n2012-07-20 14:51:45 Experiment started\n\n2012-07-20 14:51:26 Experiment ended\n\n2012-07-20 14:51:12 Experiment started\n\n2012-07-20 14:51:03 Experiment ended\n\n2012-07-20 14:50:46 Experiment started\n\n2012-07-20 14:50:35 Experiment ended\n\n2012-07-20 14:50:20 Experiment started\n\n2012-07-20 14:49:35 Experiment ended\n\n2012-07-20 14:49:12 Experiment started\n\n2012-07-20 14:41:41 Experiment ended\n\n2012-07-20 14:41:36 Experiment started\n\n2012-07-20 14:41:31 Experiment ended\n\n2012-07-20 14:41:26 Experiment started\n\n2012-07-20 14:41:22 Experiment ended\n\n2012-07-20 14:41:18 Experiment started\n\n2012-07-20 14:41:14 Experiment ended\n\n2012-07-20 14:41:10 Experiment started\n\n2012-07-20 14:38:27 Experiment ended\n\n2012-07-20 14:38:23 Experiment started\n\n2012-07-20 14:38:21 Experiment ended\n\n2012-07-20 14:36:44 Experiment started\n\n2012-07-20 14:36:40 Experiment ended\n\n2012-07-20 14:36:35 Experiment started\n\n2012-07-20 14:36:29 Experiment ended\n\n2012-07-20 14:36:25 Experiment started\n\n2012-07-20 14:36:22 Experiment ended\n\n2012-07-20 14:36:18 Experiment started\n\n2012-07-20 14:36:10 Experiment ended\n\n2012-07-20 14:36:05 Experiment started\n\n2012-07-20 14:35:41 Experiment ended\n\n2012-07-20 14:35:37 Experiment started\n\n2012-07-20 14:35:30 Experiment ended\n\n2012-07-20 14:35:25 Experiment started\n\n2012-07-20 14:35:19 Experiment ended\n\n2012-07-20 14:35:15 Experiment started\n\n2012-07-20 14:34:55 Experiment ended\n\n2012-07-20 14:34:50 Experiment started\n\n2012-07-20 14:34:30 Experiment ended\n\n2012-07-20 14:34:25 Experiment started\n\n2012-07-20 14:34:22 Experiment ended\n\n2012-07-20 14:34:18 Experiment started\n\n2012-07-20 14:34:11 Experiment ended\n\n2012-07-20 14:34:06 Experiment started\n\n2012-07-20 14:33:55 Experiment ended\n\n2012-07-20 14:33:50 Experiment started\n\n2012-07-20 12:45:25 \n\nError cleared and continued by user\n\n2012-07-20 12:45:22 Error -301707 occurred at NI-845x SPI Run Script.vi:6\r\n\r\nPossible reason(s):\n\r\nNI-845x:  The connection for the given device handle has been lost.\n\n"
  in  "Variable Actions":T1
  in  "Variable Settings":T2={"Measurements per Iteration"=1, "Local Data Path"=path "C:/Users/QCC/Documents/Cesium_project/LabVIEW Projects/data", "Experiment description suffix for filename (no spaces please)"="_100ms_PGCreadout_500", "Network Data Path"=path "Z:/", "Copy data to network"=FALSE, "Measurement Timeout (ms)"=3000.0, "Variables"=[{"Description"="compression time", "Name (a,a0...a9)"="x", "min"=0.0, "max"=0.0, "# steps"=1}, {"Description"="time delay", "Name (a,a0...a9)"="y", "min"=0.0, "max"=0.0, "# steps"=1}, {"Description"="pgc time", "Name (a,a0...a9)"="z", "min"=10.0, "max"=10.0, "# steps"=1}], "Parameters"=[{"Description"="exposure time (s)*", "Name (a,a0...a9)"="x3", "Equation"=".1", "Result"=0.1}, {"Description"="speed of light", "Name (a,a0...a9)"="c0", "Equation"="299792458", "Result"=299792458.0}, {"Description"="pi", "Name (a,a0...a9)"="z0", "Equation"="3.141592654", "Result"=3.141592654}, {"Description"="saturation intensity", "Name (a,a0...a9)"="x9", "Equation"="27", "Result"=27.0}, {"Description"="epsilon0", "Name (a,a0...a9)"="z1", "Equation"="1/(4*z0*10^(-7)*c0^2)", "Result"=8.854187816464273e-12}, {"Description"="6p3/2 gamma", "Name (a,a0...a9)"="y9", "Equation"="2*z0*5.1*10^6", "Result"=32044245.070799995}, {"Description"="kB (SI)", "Name (a,a0...a9)"="y0", "Equation"="1.38065*10^(-23)", "Result"=1.3806499999999997e-23}, {"Description"="alpha780 (cgs)", "Name (a,a0...a9)"="z2", "Equation"="-247. * 10^(-24)", "Result"=-2.4699999999999998e-22}, {"Description"="alpha 780 (SI)", "Name (a,a0...a9)"="z3", "Equation"="z2*4*z0*z1*10^(-6)", "Result"=-2.748245638452437e-38}, {"Description"="array trap spacing (d microns)", "Name (a,a0...a9)"="z4", "Equation"="3.8", "Result"=3.8}, {"Description"="array beam waist (w0 microns)", "Name (a,a0...a9)"="z5", "Equation"="1.73", "Result"=1.73}, {"Description"="array ratio (s=d/w)", "Name (a,a0...a9)"="z6", "Equation"="z4/z5", "Result"=2.1965317919075145}, {"Description"="780 power out of the fiber (W)*", "Name (a,a0...a9)"="b4", "Equation"="2.02", "Result"=2.02}, {"Description"="total power at atoms (W) ", "Name (a,a0...a9)"="z7", "Equation"="b4/2", "Result"=1.01}, {"Description"="number of array spots (n)", "Name (a,a0...a9)"="z8", "Equation"="16", "Result"=16.0}, {"Description"="peak intensity in one spot (P0)", "Name (a,a0...a9)"="z9", "Equation"="(2.*z7/z8)/(z0*z5^2 * 10^(-12))", "Result"=13427319030.190212}, {"Description"="trap depth (mK)", "Name (a,a0...a9)"="y1", "Equation"="-(0.001*2*z0*z2/(y0*c0))*z9*2*exp(-z6^2/2)*(1-4*exp(-z6^2/2))", "Result"=0.578853669827579}, {"Description"="readout detuning (MHz)*", "Name (a,a0...a9)"="y2", "Equation"="36", "Result"=36.0}, {"Description"="readout detuning", "Name (a,a0...a9)"="b3", "Equation"="y2*2*z0*10^6", "Result"=226194671.088}, {"Description"="mot beam waist 1 (mm)", "Name (a,a0...a9)"="y3", "Equation"="2.5", "Result"=2.5}, {"Description"="mot beam waist 2 (mm)", "Name (a,a0...a9)"="y4", "Equation"="2.5", "Result"=2.5}, {"Description"="mot beam waist 3 (mm)", "Name (a,a0...a9)"="y5", "Equation"="2.5", "Result"=2.5}, {"Description"="readout beam power 1 (uW)*", "Name (a,a0...a9)"="y6", "Equation"="185", "Result"=185.0}, {"Description"="readout  beam power 2 (uW)*", "Name (a,a0...a9)"="y7", "Equation"="82", "Result"=82.0}, {"Description"="readout beam power 3 (uW)*", "Name (a,a0...a9)"="y8", "Equation"="115", "Result"=115.0}, {"Description"="readout beam intensity 1", "Name (a,a0...a9)"="a0", "Equation"="2*y6*10^(-6)/(z0*y3^2*10^(-6))", "Result"=18.8439452596199}, {"Description"="readout beam intensity 2", "Name (a,a0...a9)"="x0", "Equation"="2*y7*10^(-6)/(z0*y4^2*10^(-6))", "Result"=8.352451412372064}, {"Description"="readout beam intensity 3", "Name (a,a0...a9)"="x1", "Equation"="2*y8*10^(-6)/(z0*y5^2*10^(-6))", "Result"=11.71380381003399}, {"Description"="total intensity", "Name (a,a0...a9)"="x2", "Equation"=" 2*a0+2*x0+2*x1", "Result"=77.82040096405191}, {"Description"="total saturation parameter", "Name (a,a0...a9)"="b4", "Equation"="x2/x9", "Result"=2.8822370727426634}, {"Description"="numerical aperture of jenoptiq", "Name (a,a0...a9)"="x4", "Equation"=".4", "Result"=0.4}, {"Description"="fractional solid angle", "Name (a,a0...a9)"="x5", "Equation"=".5*(1-sqrt(1-x4^2))", "Result"=0.041742430504416006}, {"Description"="transmission efficiency", "Name (a,a0...a9)"="x6", "Equation"=".8", "Result"=0.8}, {"Description"="quantum efficiency\n", "Name (a,a0...a9)"="x7", "Equation"=".7", "Result"=0.7}, {"Description"="scattering rate", "Name (a,a0...a9)"="x8", "Equation"="(y9/2)*(x2/x9)/(1+(4*b3^2)/(y9^2)+(x2/x9))", "Result"=227272.55825754048}, {"Description"="detected scattering rate for single atom", "Name (a,a0...a9)"="a1", "Equation"="x8*x5*x6*x7", "Result"=5312.669022430684}, {"Description"="detected photon number during exposure time", "Name (a,a0...a9)"="a2", "Equation"="a1*x3", "Result"=531.2669022430684}, {"Description"="conversion factor for camera (electrons/count)", "Name (a,a0...a9)"="a3", "Equation"="5.8", "Result"=5.8}, {"Description"="analog gain*", "Name (a,a0...a9)"="a4", "Equation"="4", "Result"=4.0}, {"Description"="EM sensitivity (as entered on camera page)*", "Name (a,a0...a9)"="a5", "Equation"="175", "Result"=175.0}, {"Description"="EM gain", "Name (a,a0...a9)"="b5", "Equation"="10^(((log(1000)-log(4))/250)*a5+log(4))", "Result"=190.8174102657344}, {"Description"="Expected Output Signal - Dark Signal", "Name (a,a0...a9)"="a6", "Equation"="a2*a4*b5*x7/a3", "Result"=48939.642835962055}, {"Description"="average background pixel value", "Name (a,a0...a9)"="a7", "Equation"="10914*(x3/.100)", "Result"=10914.0}, {"Description"="roi area*", "Name (a,a0...a9)"="a8", "Equation"="16", "Result"=16.0}, {"Description"="Expected Output Signal", "Name (a,a0...a9)"="a9", "Equation"="a6+a7*a8", "Result"=223563.64283596206}, {"Description"="imaging system mag", "Name (a,a0...a9)"="b0", "Equation"="25.5", "Result"=25.5}, {"Description"="camera pixel size (um)", "Name (a,a0...a9)"="b1", "Equation"="16", "Result"=16.0}, {"Description"="pixel size after mag (um)", "Name (a,a0...a9)"="b2", "Equation"="b1/b0", "Result"=0.6274509803921569}, {"Description"="gaussian point spread deterimed by airforce chart (pixels)", "Name (a,a0...a9)"="b6", "Equation"=".86", "Result"=0.86}, {"Description"="gaussian point spread (um)", "Name (a,a0...a9)"="b7", "Equation"="b2*b6", "Result"=0.5396078431372549}, {"Description"="lattice period (in pixels)", "Name (a,a0...a9)"="b8", "Equation"="z4/b2", "Result"=6.0562499999999995}], "Run Test Mode"=TRUE} {"Variables"."# steps" min=1 step=1; "Measurements per Iteration" min=1 step=1}
  out "DDS Initialized":bool=TRUE
  in  "Initialize DDS Boxes":bool
  in  "DDS Box Select Tabs":enum32{"DDS Box 1", "DDS Box 2", "DDS Errors"}(tab)
  in  "DDS Settings Box 1":T3={"DDS Profile #"=0, "RAM Mode"=[[enum."Ramp Up", enum."Direct Switch", enum."Direct Switch", enum."Ramp Up", enum."Direct Switch", enum."Direct Switch", enum."Direct Switch", enum."Direct Switch"], [enum."Direct Switch", enum."Direct Switch", enum."Direct Switch", enum."Direct Switch", enum."Direct Switch", enum."Direct Switch", enum."Direct Switch", enum."Direct Switch"], [enum."Direct Switch", enum."Direct Switch", enum."Direct Switch", enum."Direct Switch", enum."Direct Switch", enum."Direct Switch", enum."Direct Switch", enum."Direct Switch"], [enum."Direct Switch", enum."Direct Switch", enum."Direct Switch", enum."Direct Switch", enum."Direct Switch", enum."Direct Switch", enum."Direct Switch", enum."Direct Switch"]], "RAM Destination"=[0, 0, 0, 0], "Zero-crossing"=[[FALSE, FALSE, FALSE, FALSE, FALSE, FALSE, FALSE, FALSE], [FALSE, FALSE, FALSE, FALSE, FALSE, FALSE, FALSE, FALSE], [FALSE, FALSE, FALSE, FALSE, FALSE, FALSE, FALSE, FALSE], [FALSE, FALSE, FALSE, FALSE, FALSE, FALSE, FALSE, FALSE]], "No Dwell High"=[[FALSE, FALSE, FALSE, FALSE, FALSE, FALSE, FALSE, FALSE], [FALSE, FALSE, FALSE, FALSE, FALSE, FALSE, FALSE, FALSE], [FALSE, FALSE, FALSE, FALSE, FALSE, FALSE, FALSE, FALSE], [FALSE, FALSE, FALSE, FALSE, FALSE, FALSE, FALSE, FALSE]], "RAM Enable"=[FALSE, FALSE, FALSE, FALSE], "RAM Default Profile"=[{"Frequency [MHz]"="20", "Amplitude [dBm]"="-15", "Phase Offset [rad]"="0"}, {"Frequency [MHz]"="", "Amplitude [dBm]"="-50", "Phase Offset [rad]"=""}, {"Frequency [MHz]"="", "Amplitude [dBm]"="-50", "Phase Offset [rad]"=""}, {"Frequency [MHz]"="", "Amplitude [dBm]"="-50", "Phase Offset [rad]"=""}], "RAM Static Array"=[[[0.0], [0.0], [0.0], [0.0]], [[0.0], [0.0], [0.0], [0.0]], [[0.0], [0.0], [0.0], [0.0]], [[0.0], [0.0], [0.0], [0.0]], [[0.0], [0.0], [0.0], [0.0]], [[0.0], [0.0], [0.0], [0.0]], [[0.0], [0.0], [0.0], [0.0]], [[0.0], [0.0], [0.0], [0.0]]], "Function/Static"=[[TRUE, FALSE, FALSE, FALSE, FALSE, FALSE, FALSE, FALSE], [TRUE, FALSE, FALSE, FALSE, FALSE, FALSE, FALSE, FALSE], [TRUE, FALSE, FALSE, FALSE, FALSE, FALSE, FALSE, FALSE], [TRUE, FALSE, FALSE, FALSE, FALSE, FALSE, FALSE, FALSE]], "Single Tone Profiles"=[[{"Frequency [MHz]"="227", "Amplitude [dBm]"="0", "Phase Offset [rad]"="0"}, {"Frequency [MHz]"="227", "Amplitude [dBm]"="-150", "Phase Offset [rad]"="0"}, {"Frequency [MHz]"="", "Amplitude [dBm]"="", "Phase Offset [rad]"="0"}, {"Frequency [MHz]"="", "Amplitude [dBm]"="0", "Phase Offset [rad]"="0"}, {"Frequency [MHz]"="0", "Amplitude [dBm]"="-50", "Phase Offset [rad]"="0"}, {"Frequency [MHz]"="0", "Amplitude [dBm]"="-50", "Phase Offset [rad]"="0"}, {"Frequency [MHz]"="0", "Amplitude [dBm]"="-50", "Phase Offset [rad]"="0"}, {"Frequency [MHz]"="0", "Amplitude [dBm]"="-50", "Phase Offset [rad]"="0"}], [{"Frequency [MHz]"="278.5", "Amplitude [dBm]"="0", "Phase Offset [rad]"="0"}, {"Frequency [MHz]"="278.5", "Amplitude [dBm]"="-23", "Phase Offset [rad]"="0"}, {"Frequency [MHz]"="278.5", "Amplitude [dBm]"="-10", "Phase Offset [rad]"="0"}, {"Frequency [MHz]"="278.5", "Amplitude [dBm]"="-10", "Phase Offset [rad]"="0"}, {"Frequency [MHz]"="60", "Amplitude [dBm]"="-50", "Phase Offset [rad]"="0"}, {"Frequency [MHz]"="70", "Amplitude [dBm]"="-50", "Phase Offset [rad]"="0"}, {"Frequency [MHz]"="80", "Amplitude [dBm]"="-50", "Phase Offset [rad]"="0"}, {"Frequency [MHz]"="90", "Amplitude [dBm]"="-50", "Phase Offset [rad]"="0"}], [{"Frequency [MHz]"="108", "Amplitude [dBm]"="0", "Phase Offset [rad]"="0"}, {"Frequency [MHz]"="95", "Amplitude [dBm]"="-7", "Phase Offset [rad]"="0"}, {"Frequency [MHz]"="90", "Amplitude [dBm]"="-150", "Phase Offset [rad]"="0"}, {"Frequency [MHz]"="95", "Amplitude [dBm]"="-6", "Phase Offset [rad]"="0"}, {"Frequency [MHz]"="0", "Amplitude [dBm]"="-50", "Phase Offset [rad]"="0"}, {"Frequency [MHz]"="0", "Amplitude [dBm]"="-50", "Phase Offset [rad]"="0"}, {"Frequency [MHz]"="0", "Amplitude [dBm]"="-50", "Phase Offset [rad]"="0"}, {"Frequency [MHz]"="0", "Amplitude [dBm]"="-50", "Phase Offset [rad]"="0"}], [{"Frequency [MHz]"="132", "Amplitude [dBm]"="0", "Phase Offset [rad]"="0"}, {"Frequency [MHz]"="75", "Amplitude [dBm]"="0", "Phase Offset [rad]"="0"}, {"Frequency [MHz]"="0", "Amplitude [dBm]"="-50", "Phase Offset [rad]"="0"}, {"Frequency [MHz]"="0", "Amplitude [dBm]"="-50", "Phase Offset [rad]"="0"}, {"Frequency [MHz]"="0", "Amplitude [dBm]"="-50", "Phase Offset [rad]"="0"}, {"Frequency [MHz]"="0", "Amplitude [dBm]"="-50", "Phase Offset [rad]"="0"}, {"Frequency [MHz]"="0", "Amplitude [dBm]"="-50", "Phase Offset [rad]"="0"}, {"Frequency [MHz]"="0", "Amplitude [dBm]"="-50", "Phase Offset [rad]"="0"}]], "Load DDS Ch 1"=FALSE, "Load DDS Ch 2"=FALSE, "Load DDS Ch 3"=FALSE, "Load DDS Ch 4"=FALSE, "DDS Power"=[TRUE, TRUE, TRUE, TRUE], "DDS box device reference"={"NI USB-8451 device reference"="USB0::0x3923::0x7166::01574F57::RAW", "DIO port"=0, "Serial Clock Rate [kHz]"=1000, "Channels Settings"=[{"Ref Clock Rate [MHz]"=1000.0, "Full Scale Output Power [dBm]"=0.0}, {"Ref Clock Rate [MHz]"=1000.0, "Full Scale Output Power [dBm]"=0.0}, {"Ref Clock Rate [MHz]"=1000.0, "Full Scale Output Power [dBm]"=0.0}, {"Ref Clock Rate [MHz]"=1000.0, "Full Scale Output Power [dBm]"=0.0}]}, "Load RAM"=FALSE, "RAM Function Settings"=[[["10*x", "1", "1", "260", "10"], ["", "", "", "", "1"], ["", "", "", "", "1"], ["", "", "", "", "1"]], [["", "", "", "", "1"], ["", "", "", "", "1"], ["", "", "", "", "1"], ["", "", "", "", "1"]], [["", "", "", "", "1"], ["", "", "", "", "1"], ["", "", "", "", "1"], ["", "", "", "", "1"]], [["10*x", "1", "1", "260", "10"], ["", "", "", "", "1"], ["", "", "", "", "1"], ["", "", "", "", "1"]], [["", "", "", "", "1"], ["", "", "", "", "1"], ["", "", "", "", "1"], ["", "", "", "", "1"]], [["", "", "", "", "1"], ["", "", "", "", "1"], ["", "", "", "", "1"], ["", "", "", "", "1"]], [["", "", "", "", "1"], ["", "", "", "", "1"], ["", "", "", "", "1"], ["", "", "", "", "1"]], [["", "", "", "", "1"], ["", "", "", "", "1"], ["", "", "", "", "1"], ["", "", "", "", "1"]]]}
  in  "DDS Settings Box 2":T3={"DDS Profile #"=0, "RAM Mode"=[[enum."Direct Switch", enum."Direct Switch", enum."Direct Switch", enum."Direct Switch", enum."Direct Switch", enum."Direct Switch", enum."Direct Switch", enum."Direct Switch"], [enum."Direct Switch", enum."Direct Switch", enum."Direct Switch", enum."Direct Switch", enum."Direct Switch", enum."Direct Switch", enum."Direct Switch", enum."Direct Switch"], [enum."Direct Switch", enum."Direct Switch", enum."Direct Switch", enum."Direct Switch", enum."Direct Switch", enum."Direct Switch", enum."Direct Switch", enum."Direct Switch"], [enum."Direct Switch", enum."Direct Switch", enum."Direct Switch", enum."Direct Switch", enum."Direct Switch", enum."Direct Switch", enum."Direct Switch", enum."Direct Switch"]], "RAM Destination"=[0, 0, 0, 0], "Zero-crossing"=[[FALSE, FALSE, FALSE, FALSE, FALSE, FALSE, FALSE, FALSE], [FALSE, FALSE, FALSE, FALSE, FALSE, FALSE, FALSE, FALSE], [FALSE, FALSE, FALSE, FALSE, FALSE, FALSE, FALSE, FALSE], [FALSE, FALSE, FALSE, FALSE, FALSE, FALSE, FALSE, FALSE]], "No Dwell High"=[[FALSE, FALSE, FALSE, FALSE, FALSE, FALSE, FALSE, FALSE], [FALSE, FALSE, FALSE, FALSE, FALSE, FALSE, FALSE, FALSE], [FALSE, FALSE, FALSE, FALSE, FALSE, FALSE, FALSE, FALSE], [FALSE, FALSE, FALSE, FALSE, FALSE, FALSE, FALSE, FALSE]], "RAM Enable"=[FALSE, FALSE, FALSE, FALSE], "RAM Default Profile"=[{"Frequency [MHz]"="", "Amplitude [dBm]"="", "Phase Offset [rad]"=""}, {"Frequency [MHz]"="", "Amplitude [dBm]"="", "Phase Offset [rad]"=""}, {"Frequency [MHz]"="", "Amplitude [dBm]"="", "Phase Offset [rad]"=""}, {"Frequency [MHz]"="", "Amplitude [dBm]"="", "Phase Offset [rad]"=""}], "RAM Static Array"=[[[0.0], [0.0], [0.0], [0.0], [0.0], [0.0], [0.0], [0.0], [0.0], [0.0], [0.0]]], "Function/Static"=[[FALSE, FALSE, FALSE, FALSE, FALSE, FALSE, FALSE, FALSE], [FALSE, FALSE, FALSE, FALSE, FALSE, FALSE, FALSE, FALSE], [FALSE, FALSE, FALSE, FALSE, FALSE, FALSE, FALSE, FALSE], [FALSE, FALSE, FALSE, FALSE, FALSE, FALSE, FALSE, FALSE]], "Single Tone Profiles"=[[{"Frequency [MHz]"="153", "Amplitude [dBm]"="0", "Phase Offset [rad]"="0"}, {"Frequency [MHz]"="157.5", "Amplitude [dBm]"="-10", "Phase Offset [rad]"="0"}, {"Frequency [MHz]"="157.5", "Amplitude [dBm]"="-22", "Phase Offset [rad]"="0"}, {"Frequency [MHz]"="157.5", "Amplitude [dBm]"="-22", "Phase Offset [rad]"="0"}, {"Frequency [MHz]"="157.5", "Amplitude [dBm]"="-22", "Phase Offset [rad]"="0"}, {"Frequency [MHz]"="157.5", "Amplitude [dBm]"="-22", "Phase Offset [rad]"="0"}, {"Frequency [MHz]"="157.5", "Amplitude [dBm]"="-22", "Phase Offset [rad]"="0"}, {"Frequency [MHz]"="157.5", "Amplitude [dBm]"="-22", "Phase Offset [rad]"="0"}], [{"Frequency [MHz]"="83", "Amplitude [dBm]"="0", "Phase Offset [rad]"="0"}, {"Frequency [MHz]"="0", "Amplitude [dBm]"="0", "Phase Offset [rad]"="0"}, {"Frequency [MHz]"="157.5", "Amplitude [dBm]"="-22", "Phase Offset [rad]"="0"}, {"Frequency [MHz]"="157.5", "Amplitude [dBm]"="-22", "Phase Offset [rad]"="0"}, {"Frequency [MHz]"="157.5", "Amplitude [dBm]"="-22", "Phase Offset [rad]"="0"}, {"Frequency [MHz]"="157.5", "Amplitude [dBm]"="-22", "Phase Offset [rad]"="0"}, {"Frequency [MHz]"="157.5", "Amplitude [dBm]"="-22", "Phase Offset [rad]"="0"}, {"Frequency [MHz]"="157.5", "Amplitude [dBm]"="-22", "Phase Offset [rad]"="0"}], [{"Frequency [MHz]"="150", "Amplitude [dBm]"="0", "Phase Offset [rad]"="0"}, {"Frequency [MHz]"="0", "Amplitude [dBm]"="0", "Phase Offset [rad]"="0"}, {"Frequency [MHz]"="157.5", "Amplitude [dBm]"="-22", "Phase Offset [rad]"="0"}, {"Frequency [MHz]"="157.5", "Amplitude [dBm]"="-22", "Phase Offset [rad]"="0"}, {"Frequency [MHz]"="157.5", "Amplitude [dBm]"="-22", "Phase Offset [rad]"="0"}, {"Frequency [MHz]"="157.5", "Amplitude [dBm]"="-22", "Phase Offset [rad]"="0"}, {"Frequency [MHz]"="157.5", "Amplitude [dBm]"="-22", "Phase Offset [rad]"="0"}, {"Frequency [MHz]"="150", "Amplitude [dBm]"="0", "Phase Offset [rad]"="0"}], [{"Frequency [MHz]"="150", "Amplitude [dBm]"="0", "Phase Offset [rad]"="0"}, {"Frequency [MHz]"="0", "Amplitude [dBm]"="0", "Phase Offset [rad]"="0"}, {"Frequency [MHz]"="157.5", "Amplitude [dBm]"="-22", "Phase Offset [rad]"="0"}, {"Frequency [MHz]"="157.5", "Amplitude [dBm]"="-22", "Phase Offset [rad]"="0"}, {"Frequency [MHz]"="157.5", "Amplitude [dBm]"="-22", "Phase Offset [rad]"="0"}, {"Frequency [MHz]"="157.5", "Amplitude [dBm]"="-22", "Phase Offset [rad]"="0"}, {"Frequency [MHz]"="157.5", "Amplitude [dBm]"="-22", "Phase Offset [rad]"="0"}, {"Frequency [MHz]"="150", "Amplitude [dBm]"="0", "Phase Offset [rad]"="0"}]], "Load DDS Ch 1"=FALSE, "Load DDS Ch 2"=FALSE, "Load DDS Ch 3"=FALSE, "Load DDS Ch 4"=FALSE, "DDS Power"=[FALSE, FALSE, TRUE, TRUE], "DDS box device reference"={"NI USB-8451 device reference"="USB0::0x3923::0x7166::01574FA5::RAW", "DIO port"=0, "Serial Clock Rate [kHz]"=1000, "Channels Settings"=[{"Ref Clock Rate [MHz]"=1000.0, "Full Scale Output Power [dBm]"=0.0}, {"Ref Clock Rate [MHz]"=1000.0, "Full Scale Output Power [dBm]"=0.0}, {"Ref Clock Rate [MHz]"=1000.0, "Full Scale Output Power [dBm]"=0.0}, {"Ref Clock Rate [MHz]"=1000.0, "Full Scale Output Power [dBm]"=0.0}]}, "Load RAM"=FALSE, "RAM Function Settings"=[[["", "", "", "", ""], ["", "", "", "", ""], ["", "", "", "", ""], ["", "", "", "", ""], ["", "", "", "", ""], ["", "", "", "", ""], ["", "", "", "", ""], ["", "", "", "", ""], ["", "", "", "", ""], ["", "", "", "", ""], ["", "", "", "", ""]]]}
  in  "Check DDS Box 2":bool
  in  "Check DDS Box 1":bool
  out "Box 1 CFR1":u8[][](array[numeric])
  out "Box 1 CFR2":u8[][](array[numeric])
  out "Box 1 CFR3":u8[][](array[numeric])
  out "Box 2 CFR1":u8[][](array[numeric])
  out "Box 2 CFR2":u8[][](array[numeric])
  out "Box 2 CFR3":u8[][](array[numeric])
  in  "Save DDS Data":bool
  in  "Load DDS Data":bool
  in  "DDS # of Boxes":i32=1 min=0 max=2 step=1
  out "DDS Coms Okay?":bool[](array[boolean])
  out "Error LED":bool caption="Error"
  # "Parameters will be evaluated once at the beginning of the experiment from top to bottom, \nso any parameter may depend on all those above it.\nVariables will be evaluated each iteration.\nParameters and Variables may be used in various other experiment settings, as noted.\nSee LabView Help -> Formula Node and Expression Node Functions for a list of available functions."
  # "Ch. 1"
  # "Ch. 2"
  # "Ch. 3"
  # "Ch. 4"
  # "Ch. 1"
  # "Ch. 2"
  # "Ch. 3"
  # "Ch. 4"
  # "Ch. 1"
  # "Ch. 2"
  # "Ch. 3"
  # "Ch. 4"
  # "Ch. 1"
  # "Ch. 2"
  # "Ch. 3"
  # "Ch. 4"
  # "Ch. 1"
  # "Ch. 2"
  # "Ch. 3"
  # "Ch. 4"
  # "Ch. 1"
  # "Ch. 2"
  # "Ch. 3"
  # "Ch. 4"
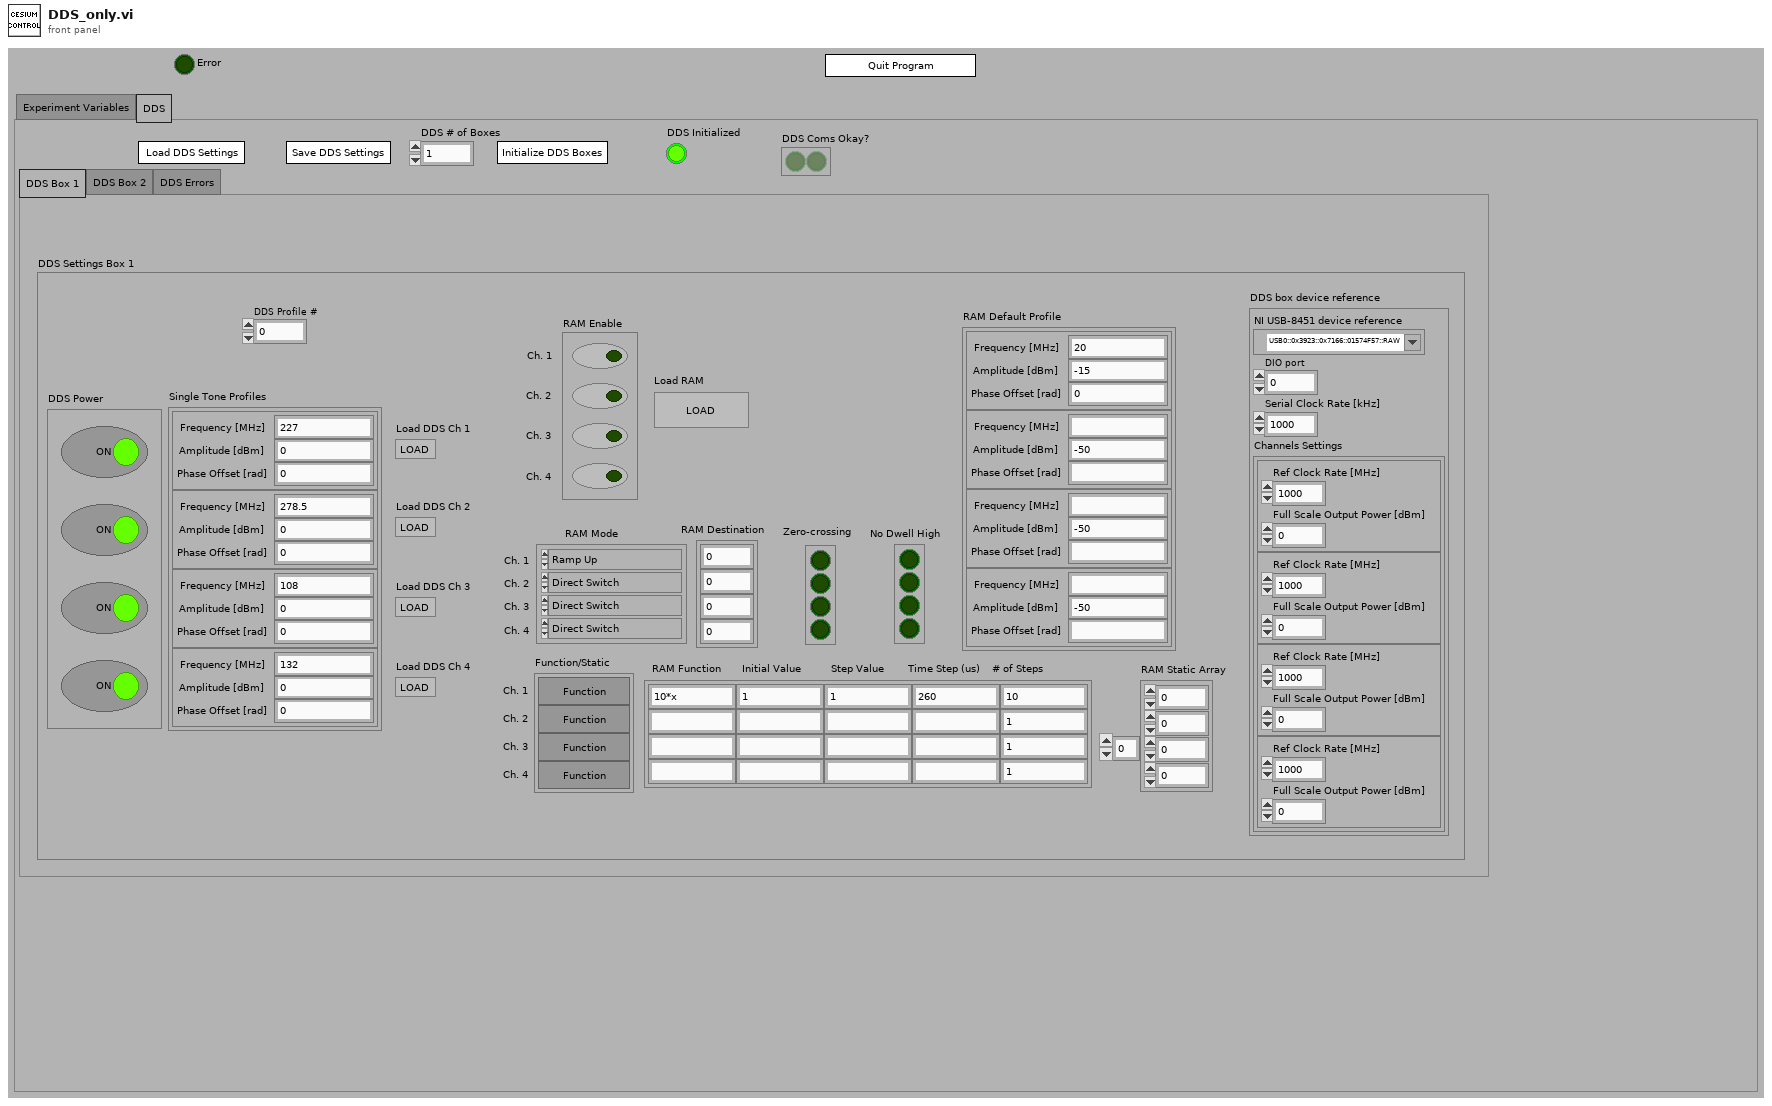
[diagram p1: front panel]
types:
  T1 = cluster{"Load All Variable Settings":bool, "Save All Variable Settings":bool, "Load Variables":bool, "Save Variables":bool, "Load Paramters":bool, "Save Parameters":bool, "Evaluate Parameters":bool, "Clear Log":bool, "Save Log":bool}
  T2 = typedef "ExperimentVariables.lvclass/Variable_Settings.ctl" = cluster{"Measurements per Iteration":i32, "Local Data Path":path, "Experiment description suffix for filename (no spaces please)":string, "Network Data Path":path, "Copy data to network":bool, "Measurement Timeout (ms)":dbl, "Variables":cluster{"Description":string, "Name (a,a0...a9)":string, "min":dbl, "max":dbl, "# steps":u32}[], "Parameters":cluster{"Description":string, "Name (a,a0...a9)":string, "Equation":string, "Result":dbl}[], "Run Test Mode":bool}
  T3 = typedef "DDS Settings.ctl" = cluster{"DDS Profile #":u8, "RAM Mode":T4[][], "RAM Destination":u8[], "Zero-crossing":bool[][], "No Dwell High":bool[][], "RAM Enable":bool[], "RAM Default Profile":cluster{"Frequency [MHz]":string, "Amplitude [dBm]":string, "Phase Offset [rad]":string}[], "RAM Static Array":dbl[][][], "Function/Static":bool[][], "Single Tone Profiles":cluster{"Frequency [MHz]":string, "Amplitude [dBm]":string, "Phase Offset [rad]":string}[][], "Load DDS Ch 1":bool, "Load DDS Ch 2":bool, "Load DDS Ch 3":bool, "Load DDS Ch 4":bool, "DDS Power":bool[], "DDS box device reference":T5, "Load RAM":bool, "RAM Function Settings":string[][][]}
  T4 = typedef "DDS RAM mode.ctl" = enum16{"Direct Switch", "Ramp Up", "Bidirectional Ramp", "Continuous Bidirectional Ramp", "Continuous Recirculate", "Direct Switch 2", "Direct Switch 3", "Direct Switch 4"}
  T5 = typedef "DDS box device reference.ctl" = cluster{"NI USB-8451 device reference":T6, "DIO port":u8, "Serial Clock Rate [kHz]":u16, "Channels Settings":cluster{"Ref Clock Rate [MHz]":dbl, "Full Scale Output Power [dBm]":dbl}[]}
  T6 = typedef "ni845xControl.ctl" = refnum<k21>
  T7 = enum16{"Append to Log", "Register Log Display Refnum", "Clear Log", "Clear Log Display Refnums"}
  T8 = typedef "DialogType.ctl" = u16
  T9 = typedef "AD9910 registers.ctl" = enum16{"CFR1", "CFR2", "CFR3", "Auxiliary DAC Control", "I/0 Update Rate", "Frequency Tuning Word", "Phase Offset Word", "Amplitude Scale Factor", "Multichip Sync", "Digital Ramp Limit", "Digital Ramp Step Size", "Digital Ramp Rate", "Single Tone Profile 0", "Single Tone Profile 1", "Single Tone Profile 2", "Single Tone Profile 3", "Single Tone Profile 4", "Single Tone Profile 5", "Single Tone Profile 6", "Single Tone Profile 7", "RAM Profile 0", "RAM Profile 1", "RAM Profile 2", "RAM Profile 3", "RAM Profile 4", "RAM Profile 5", "RAM Profile 6", "RAM Profile 7", "RAM"}
  T10 = cluster{"Description":string, "Name (a,a0...a9)":string, "min":dbl, "max":dbl, "# steps":u32}
  T11 = cluster{"Description":string, "Name (a,a0...a9)":string, "Equation":string, "Result":dbl}
  T12 = cluster{"Description":string, "Name (a,a0...a9)":string, "min":dbl, "max":dbl, "# steps":u32}[]
  T13 = cluster{"Description":string, "Name (a,a0...a9)":string, "Equation":string, "Result":dbl}[]
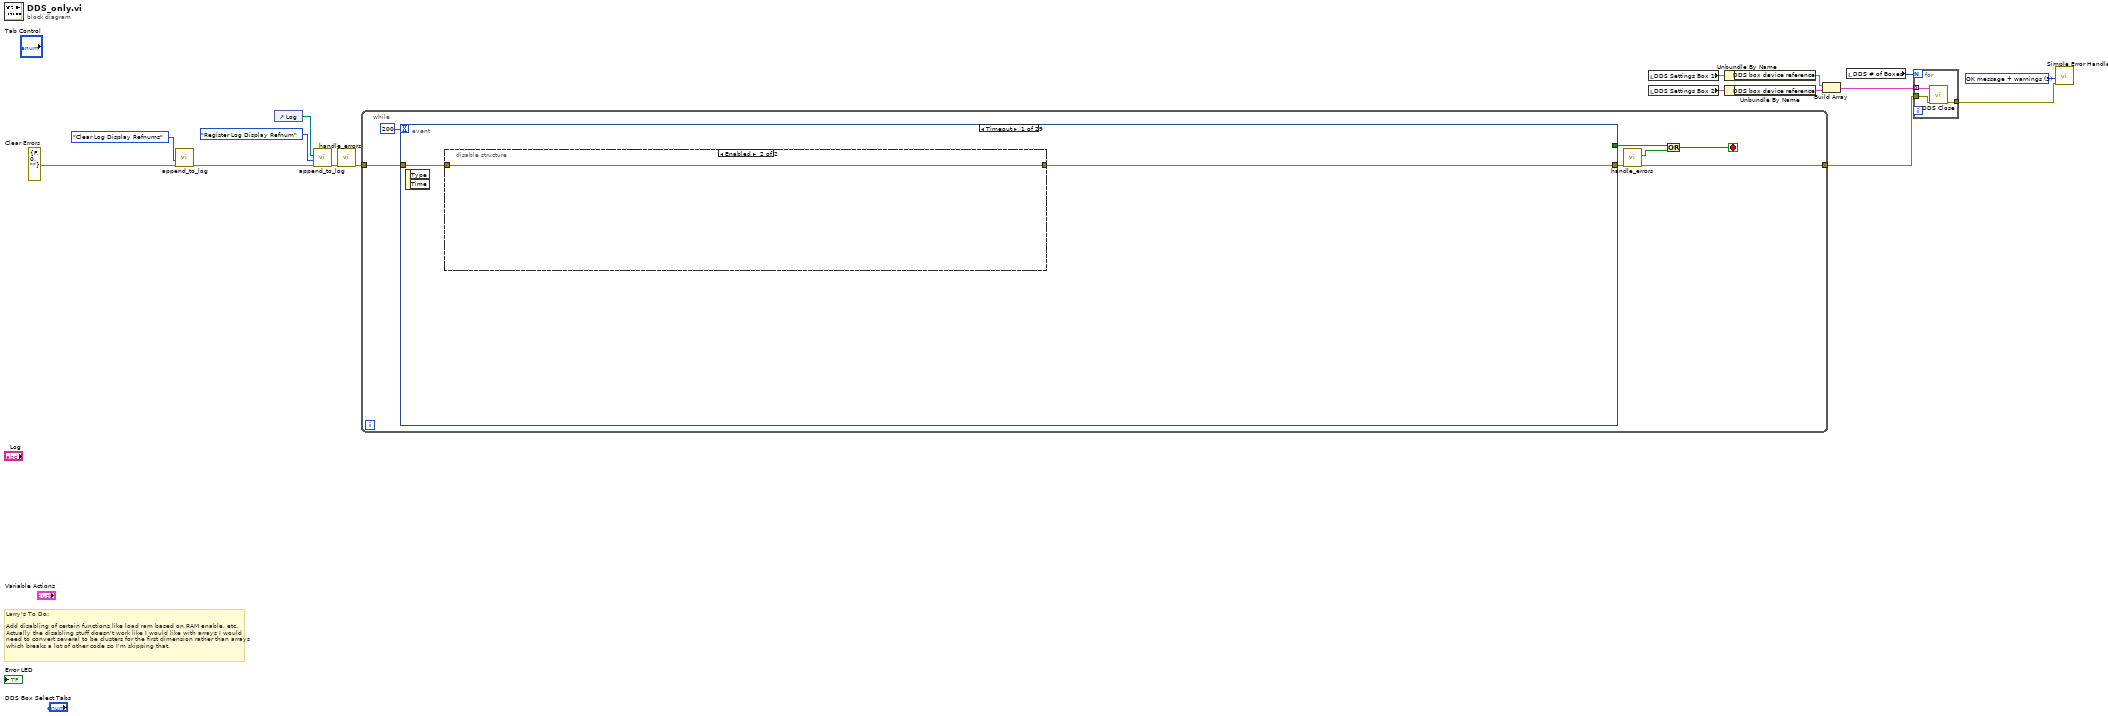
[diagram p0: block diagram]
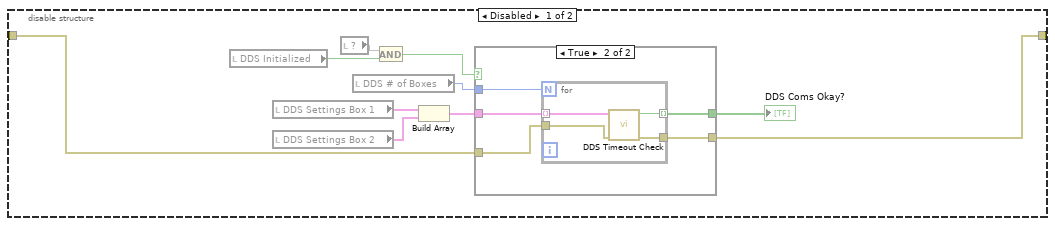
[diagram p2: hidden frame]
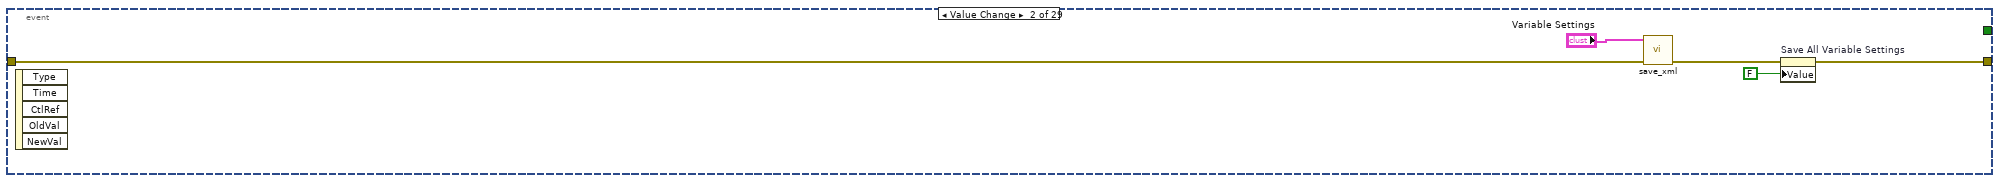
[diagram p4: hidden frame]
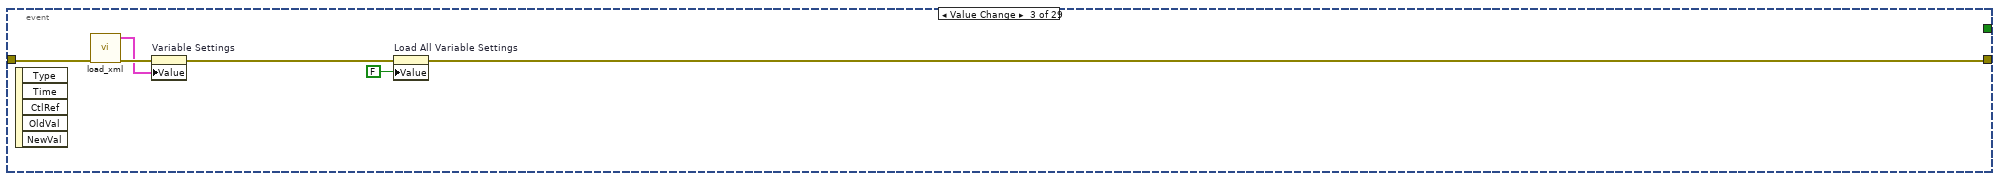
[diagram p5: hidden frame]
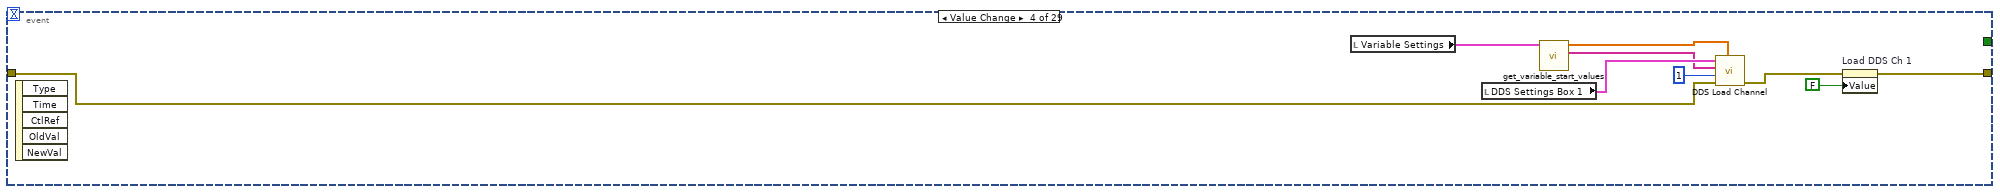
[diagram p6: hidden frame]
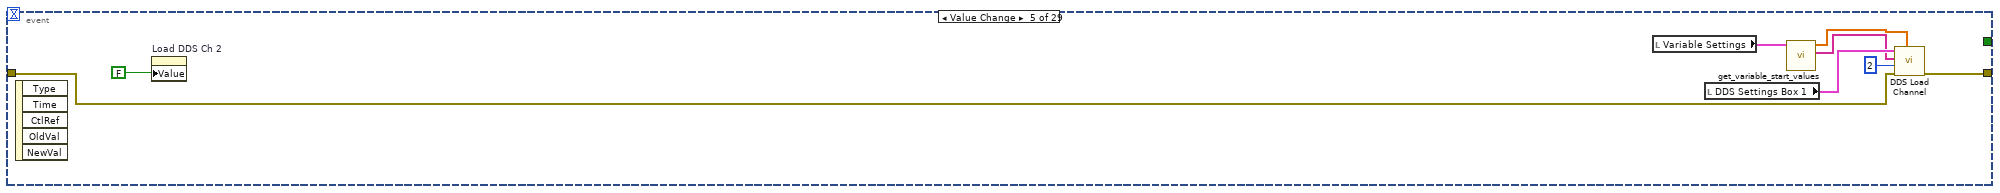
[diagram p7: hidden frame]
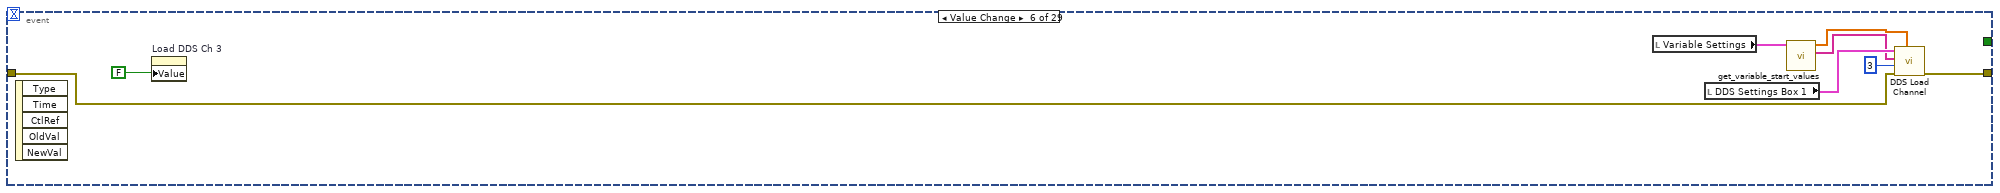
[diagram p8: hidden frame]
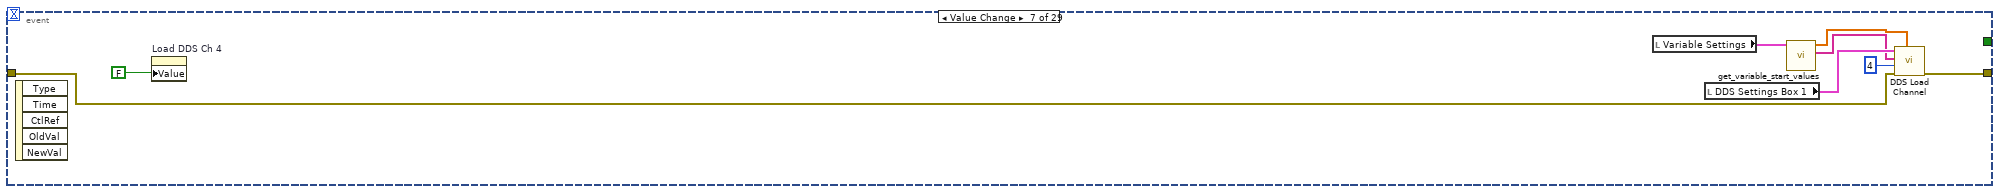
[diagram p9: hidden frame]
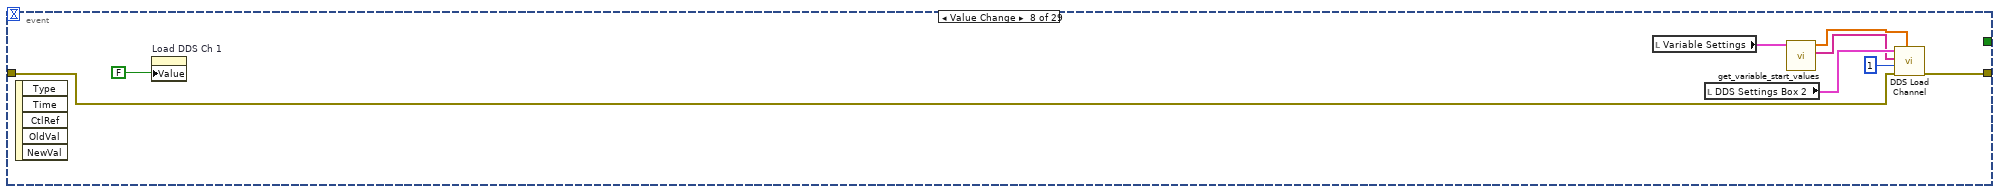
[diagram p10: hidden frame]
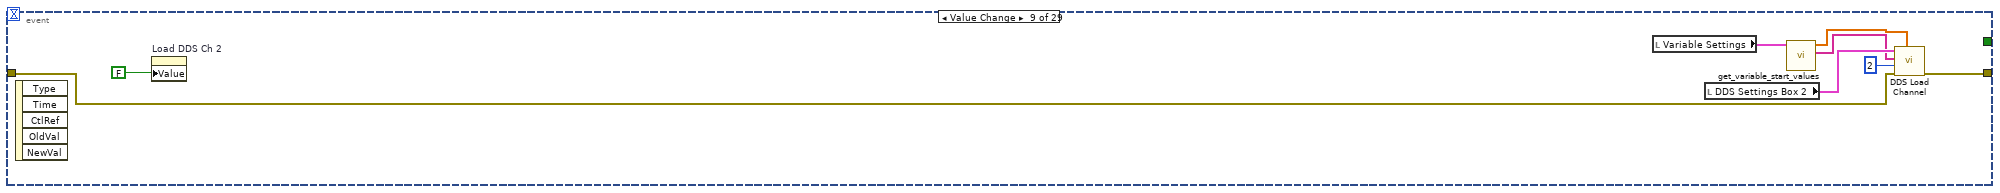
[diagram p11: hidden frame]
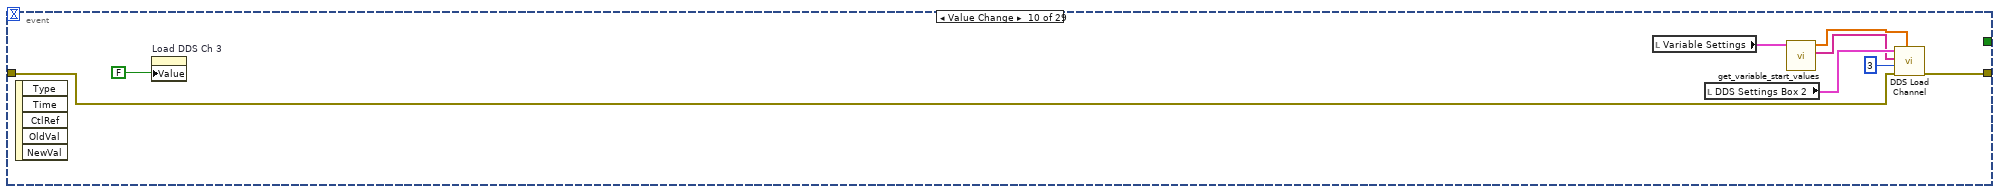
[diagram p12: hidden frame]
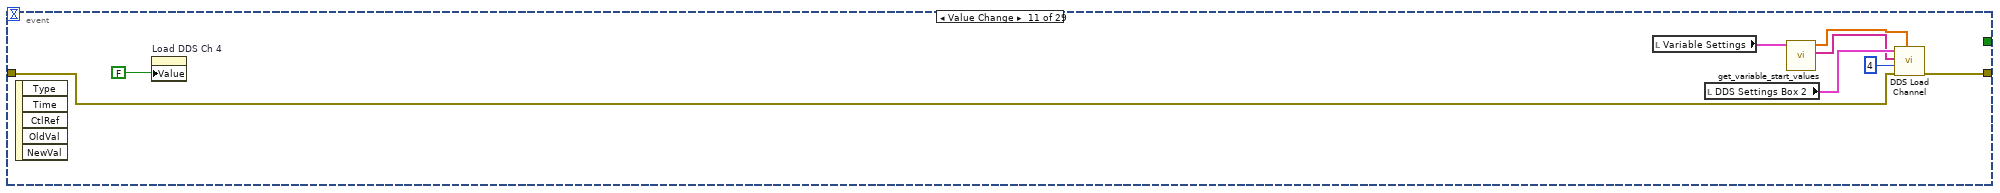
[diagram p13: hidden frame]
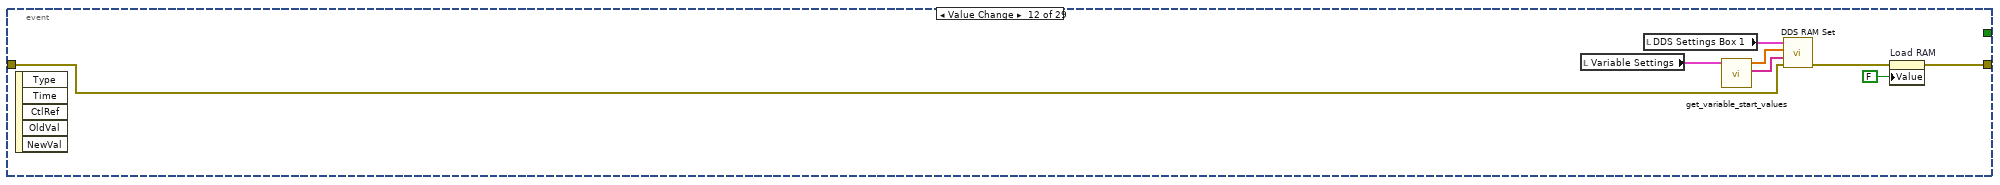
[diagram p14: hidden frame]
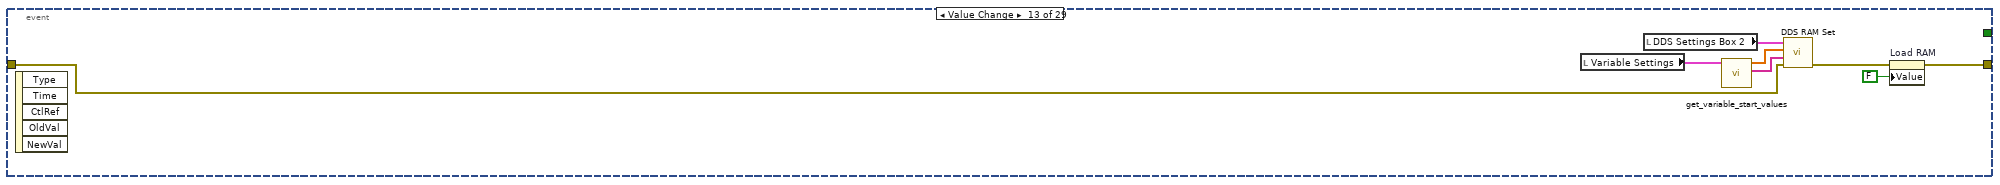
[diagram p15: hidden frame]
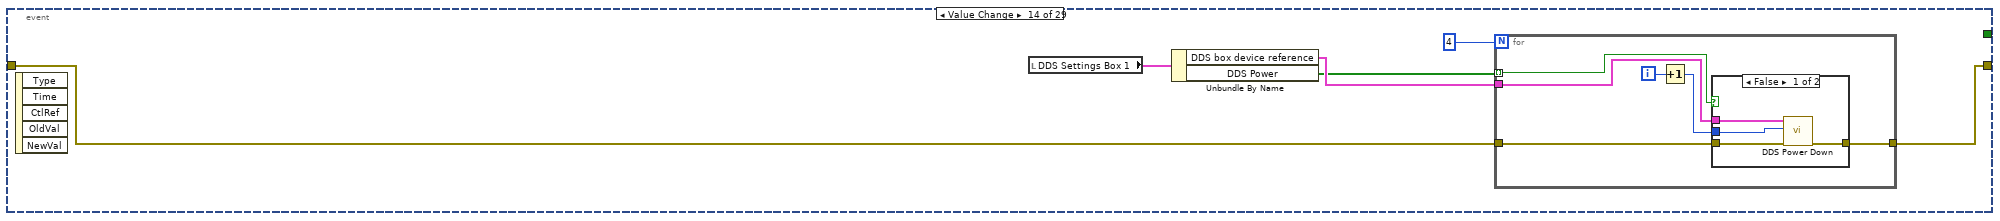
[diagram p16: hidden frame]
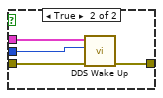
[diagram p17: hidden frame]
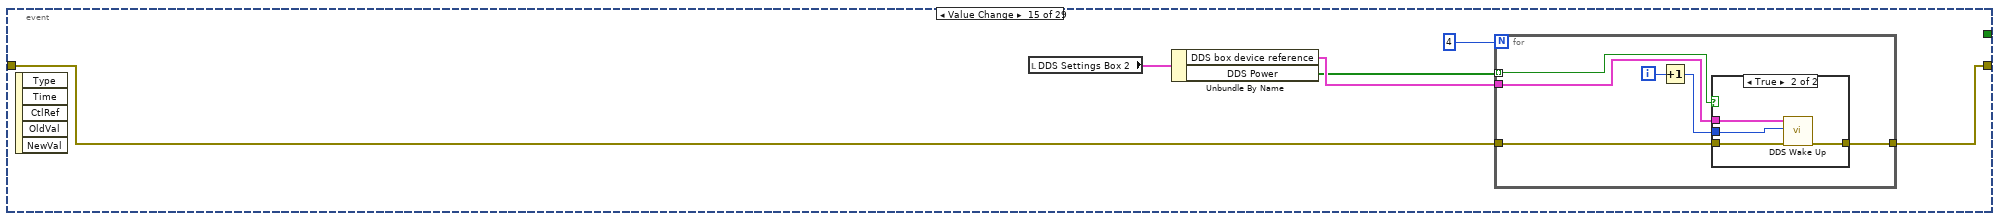
[diagram p18: hidden frame]
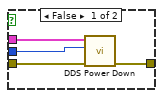
[diagram p19: hidden frame]
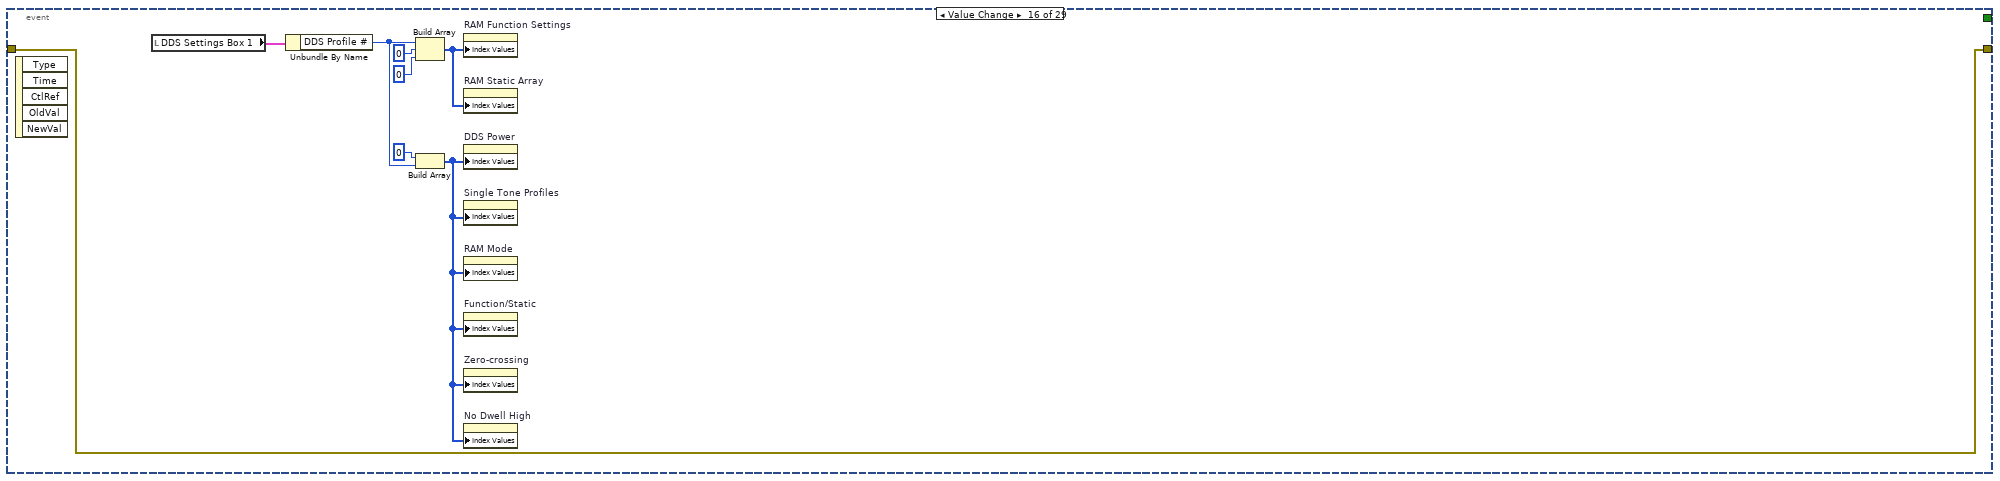
[diagram p20: hidden frame]
diagram:
  w16 = T8 3 items=["no dialog", "OK message", "continue or stop message", "OK message + warnings", "continue/stop + warnings"] ("type of dialog (OK msg:1)")
  w1 = errorcluster {"status"=FALSE, "code"=0, "source"=""}  # Clear Errors
  # "Larry's To Do:\n\nAdd disabling of certain functions like load ram based on RAM enable, etc.\nActually the disabling stuff doesn't work like I would like with arrays I would \nneed to convert several to be clusters for the first dimension rather than arrays\nwhich breaks a lot of other code so I'm skipping that."
  n1 = call "append_to_log.vi"("error in"=w1, "Action"=T7."Clear Log Display Refnums") -> ("error out"=w11:errorcluster)  [unwired: 9 in]
  n2 = control-ref of="Log"() -> (w9:refnum<vi>)
  n3 = call "append_to_log.vi"("error in"=w11, "Action"=T7."Register Log Display Refnum", "Log (String) Refnum (in)"=w9) -> ("error out"=w10:errorcluster)  [unwired: 8 in]
  n4 = call "handle_errors.vi"("error in (no error)"=w10) -> ("error out"=w12:errorcluster)  [unwired: 9 in, 1 out]
  n5 = while {
    tunnel: w12 -> [w22]
    tunnel: [w18] -> w15
    stop <- w21 stop-if-true
    n6 = event shown="[0] Timeout" {
      selector: _ -> [_ _ _ _ _ _ _ _ _ _ _ _ _ _ _ _ _ _ _ _ _ _ _ _ _ _ _ _ _]
      dyn-events: _ -> [_ _ _ _ _ _ _ _ _ _ _ _ _ _ _ _ _ _ _ _ _ _ _ _ _ _ _ _ _]
      timeout: 200 -> [_ _ _ _ _ _ _ _ _ _ _ _ _ _ _ _ _ _ _ _ _ _ _ _ _ _ _ _ _]
      tunnel: w22 -> [w24 w49 w55 w64 w71 w79 w87 w96 w104 w112 w120 w130 w138 w141 w161 w186 w191 w198 w218 w244 w271 w290 w296 w301 w309 w325 w346 w353 w358]
      tunnel: [w25 w51 w57 w61 w70 w80 w86 w94 w102 w110 w119 w126 w131 w140 w159 w186 w191 w193 w217 w252 w276 w291 w298 w299 w311 w324 w343 w352 w358] -> w20
      tunnel: [_ _ _ _ _ _ _ _ _ _ _ _ _ _ _ _ _ _ _ _ _ _ _ _ _ _ _ _ TRUE] -> w19
      event Timeout {
        n7 = event-data() -> ()  [unwired: 1 in, 2 out]
        n8 = disable-structure shown="Enabled" {
          disable-tunnel: [w35 w46] -> w25
          disable-tunnel: w24 -> [w26 w46]
          frame Disabled {
            n9 = local read "DDS Initialized"() -> (w29:bool)
            n10 = local read "DDS Settings Box 1"() -> (w34:T3)
            n11 = local read "DDS Settings Box 2"() -> (w33:T3)
            n12 = local read item#-1() -> (w28)
            n13 = local read "DDS # of Boxes"() -> (w31:i32)
            n14 = And(x=w28, y=w29) -> (x .and. y?=w27:bool)
            n15 = Build Array(w34, w33) -> (w32:T3[])
            n16 = case shown="True" w27 {
              tunnel: w32 -> [_ w41]
              tunnel: w31 -> [_ w40]
              tunnel: w26 -> [w36 w39]
              tunnel: [_ w38] -> w30
              tunnel: [w36 w37] -> w35
              frame False {
              }
              frame True {
                n17 = for {
                  N: w40 -> [_]
                  tunnel: w41 -> [w43] mode=indexing
                  tunnel: w39 -> [w45]
                  tunnel: [w44] -> w38 mode=indexing
                  tunnel: [w42] -> w37
                  n18 = call "DDS Timeout Check.vi"("error in (no error)"=w45, "DDS Settings Box"=w43) -> ("error out"=w42:errorcluster, "DDS Comms OK?"=w44:bool)  [unwired: 8 in]
                }
              }
            }
            "DDS Coms Okay?" <- w30
          }
          frame Enabled {
          }
        }
      }
      event "Variable Actions.Save All Variable Settings": Value Change {
        n19 = event-data() -> ()  [unwired: 1 in, 5 out]
        n20 = call "save_xml.vi"("error in"=w49, "Variable Settings"="Variable Settings") -> ("error out"=w48:errorcluster)  [unwired: 9 in]
        n21 = property on="Save All Variable Settings" class="Bool (strict)"(error in=w48, "Value"=FALSE) -> (error out=w51:errorcluster)  [unwired: 1 in, 1 out]
      }
      event "Variable Actions.Load All Variable Settings": Value Change {
        n22 = event-data() -> ()  [unwired: 1 in, 5 out]
        n23 = call "load_xml.vi"("error in"=w55) -> ("error out"=w54:errorcluster, "Variable Settings"=w53:T2)  [unwired: 9 in]
        n24 = property on="Variable Settings" class="Clust (strict)"(error in=w54, "Value"=w53) -> (error out=w52:errorcluster)  [unwired: 1 in, 1 out]
        n25 = property on="Load All Variable Settings" class="Bool (strict)"(error in=w52, "Value"=FALSE) -> (error out=w57:errorcluster)  [unwired: 1 in, 1 out]
      }
      event Value Change {
        n26 = event-data() -> ()  [unwired: 1 in, 5 out]
        n27 = local read "Variable Settings"() -> (w60:T2)
        n28 = local read "DDS Settings Box 1"() -> (w65:T3)
        n29 = call "get_variable_start_values.vi"("Variable Settings"=w60) -> ("variable/parameter names"=w59:string[], "minimum/current values"=w58:dbl[])  [unwired: 9 in]
        n30 = call "DDS Load Channel.vi"("variable/parameter values"=w58, "error in"=w64, "chanel number"=u8 1 ("chanel number (1)"), "variable/parameter names"=w59, "DDS Settings Box"=w65) -> ("error out"=w62:errorcluster)  [unwired: 6 in]
        n31 = property on="Load DDS Ch 1" class="Bool (strict)"(error in=w62, "Value"=FALSE) -> (error out=w61:errorcluster)  [unwired: 1 in, 1 out]
      }
      event Value Change {
        n32 = event-data() -> ()  [unwired: 1 in, 5 out]
        n33 = property on="Load DDS Ch 2" class="Bool (strict)"("Value"=FALSE) -> ()  [unwired: 2 in, 2 out]
        n34 = local read "Variable Settings"() -> (w69:T2)
        n35 = local read "DDS Settings Box 1"() -> (w73:T3)
        n36 = call "get_variable_start_values.vi"("Variable Settings"=w69) -> ("variable/parameter names"=w68:string[], "minimum/current values"=w67:dbl[])  [unwired: 9 in]
        n37 = call "DDS Load Channel.vi"("variable/parameter values"=w67, "error in"=w71, "chanel number"=u8 2, "variable/parameter names"=w68, "DDS Settings Box"=w73) -> ("error out"=w70:errorcluster)  [unwired: 6 in]
      }
      event Value Change {
        n38 = event-data() -> ()  [unwired: 1 in, 5 out]
        n39 = property on="Load DDS Ch 3" class="Bool (strict)"("Value"=FALSE) -> ()  [unwired: 2 in, 2 out]
        n40 = local read "Variable Settings"() -> (w77:T2)
        n41 = local read "DDS Settings Box 1"() -> (w81:T3)
        n42 = call "get_variable_start_values.vi"("Variable Settings"=w77) -> ("variable/parameter names"=w76:string[], "minimum/current values"=w75:dbl[])  [unwired: 9 in]
        n43 = call "DDS Load Channel.vi"("variable/parameter values"=w75, "error in"=w79, "chanel number"=u8 3, "variable/parameter names"=w76, "DDS Settings Box"=w81) -> ("error out"=w80:errorcluster)  [unwired: 6 in]
      }
      event Value Change {
        n44 = event-data() -> ()  [unwired: 1 in, 5 out]
        n45 = property on="Load DDS Ch 4" class="Bool (strict)"("Value"=FALSE) -> ()  [unwired: 2 in, 2 out]
        n46 = local read "Variable Settings"() -> (w85:T2)
        n47 = local read "DDS Settings Box 1"() -> (w89:T3)
        n48 = call "get_variable_start_values.vi"("Variable Settings"=w85) -> ("variable/parameter names"=w84:string[], "minimum/current values"=w83:dbl[])  [unwired: 9 in]
        n49 = call "DDS Load Channel.vi"("variable/parameter values"=w83, "error in"=w87, "chanel number"=u8 4, "variable/parameter names"=w84, "DDS Settings Box"=w89) -> ("error out"=w86:errorcluster)  [unwired: 6 in]
      }
      event Value Change {
        n50 = event-data() -> ()  [unwired: 1 in, 5 out]
        n51 = property on="Load DDS Ch 1" class="Bool (strict)"("Value"=FALSE) -> ()  [unwired: 2 in, 2 out]
        n52 = local read "Variable Settings"() -> (w93:T2)
        n53 = local read "DDS Settings Box 2"() -> (w97:T3)
        n54 = call "get_variable_start_values.vi"("Variable Settings"=w93) -> ("variable/parameter names"=w91:string[], "minimum/current values"=w92:dbl[])  [unwired: 9 in]
        n55 = call "DDS Load Channel.vi"("variable/parameter values"=w92, "error in"=w96, "chanel number"=u8 1, "variable/parameter names"=w91, "DDS Settings Box"=w97) -> ("error out"=w94:errorcluster)  [unwired: 6 in]
      }
      event Value Change {
        n56 = event-data() -> ()  [unwired: 1 in, 5 out]
        n57 = property on="Load DDS Ch 2" class="Bool (strict)"("Value"=FALSE) -> ()  [unwired: 2 in, 2 out]
        n58 = local read "Variable Settings"() -> (w101:T2)
        n59 = local read "DDS Settings Box 2"() -> (w105:T3)
        n60 = call "get_variable_start_values.vi"("Variable Settings"=w101) -> ("variable/parameter names"=w99:string[], "minimum/current values"=w100:dbl[])  [unwired: 9 in]
        n61 = call "DDS Load Channel.vi"("variable/parameter values"=w100, "error in"=w104, "chanel number"=u8 2, "variable/parameter names"=w99, "DDS Settings Box"=w105) -> ("error out"=w102:errorcluster)  [unwired: 6 in]
      }
      event Value Change {
        n62 = event-data() -> ()  [unwired: 1 in, 5 out]
        n63 = property on="Load DDS Ch 3" class="Bool (strict)"("Value"=FALSE) -> ()  [unwired: 2 in, 2 out]
        n64 = local read "Variable Settings"() -> (w109:T2)
        n65 = local read "DDS Settings Box 2"() -> (w113:T3)
        n66 = call "get_variable_start_values.vi"("Variable Settings"=w109) -> ("variable/parameter names"=w108:string[], "minimum/current values"=w107:dbl[])  [unwired: 9 in]
        n67 = call "DDS Load Channel.vi"("variable/parameter values"=w107, "error in"=w112, "chanel number"=u8 3, "variable/parameter names"=w108, "DDS Settings Box"=w113) -> ("error out"=w110:errorcluster)  [unwired: 6 in]
      }
      event Value Change {
        n68 = event-data() -> ()  [unwired: 1 in, 5 out]
        n69 = property on="Load DDS Ch 4" class="Bool (strict)"("Value"=FALSE) -> ()  [unwired: 2 in, 2 out]
        n70 = local read "Variable Settings"() -> (w117:T2)
        n71 = local read "DDS Settings Box 2"() -> (w121:T3)
        n72 = call "get_variable_start_values.vi"("Variable Settings"=w117) -> ("variable/parameter names"=w116:string[], "minimum/current values"=w115:dbl[])  [unwired: 9 in]
        n73 = call "DDS Load Channel.vi"("variable/parameter values"=w115, "error in"=w120, "chanel number"=u8 4, "variable/parameter names"=w116, "DDS Settings Box"=w121) -> ("error out"=w119:errorcluster)  [unwired: 6 in]
      }
      event Value Change {
        n74 = event-data() -> ()  [unwired: 1 in, 5 out]
        n75 = local read "Variable Settings"() -> (w125:T2)
        n76 = local read "DDS Settings Box 1"() -> (w129:T3)
        n77 = call "get_variable_start_values.vi"("Variable Settings"=w125) -> ("variable/parameter names"=w123:string[], "minimum/current values"=w124:dbl[])  [unwired: 9 in]
        n78 = call "DDS RAM Set.vi"("error in (no error)"=w130, "Variable Names"=w123, "Variable Values"=w124, "DDS RAM Settings"=w129) -> ("error out"=w127:errorcluster)  [unwired: 6 in, 1 out]
        n79 = property on="Load RAM" class="Bool (strict)"(error in=w127, "Value"=FALSE) -> (error out=w126:errorcluster)  [unwired: 1 in, 1 out]
      }
      event Value Change {
        n80 = event-data() -> ()  [unwired: 1 in, 5 out]
        n81 = local read "Variable Settings"() -> (w133:T2)
        n82 = local read "DDS Settings Box 2"() -> (w137:T3)
        n83 = call "get_variable_start_values.vi"("Variable Settings"=w133) -> ("variable/parameter names"=w134:string[], "minimum/current values"=w135:dbl[])  [unwired: 9 in]
        n84 = call "DDS RAM Set.vi"("error in (no error)"=w138, "Variable Names"=w134, "Variable Values"=w135, "DDS RAM Settings"=w137) -> ("error out"=w132:errorcluster)  [unwired: 6 in, 1 out]
        n85 = property on="Load RAM" class="Bool (strict)"(error in=w132, "Value"=FALSE) -> (error out=w131:errorcluster)  [unwired: 1 in, 1 out]
      }
      event Value Change {
        n86 = event-data() -> ()  [unwired: 1 in, 5 out]
        n87 = local read "DDS Settings Box 1"() -> (w139:T3)
        n88 = Unbundle By Name(w139) -> ("DDS box device reference"=w143:T5, "DDS Power"=w142:bool[])
        n89 = for {
          N: 4 -> [_]
          tunnel: w143 -> [w148]
          tunnel: w142 -> [w147] mode=indexing
          tunnel: w141 -> [w146]
          tunnel: [w145] -> w140
          i -> [w150]
          n90 = Increment(x=w150) -> (x+1=w149:i32)
          n91 = case shown="False" w147 {
            tunnel: w149 -> [w154 w158]
            tunnel: w148 -> [w153 w157]
            tunnel: w146 -> [w152 w156]
            tunnel: [w151 w155] -> w145
            frame False {
              n92 = call "DDS Power Down.vi"("error in (no error)"=w152, "chanel number (1)"=w154, "DDS ref in"=w153) -> ("error out"=w151:errorcluster)  [unwired: 7 in, 1 out]
            }
            frame True {
              n93 = call "DDS Wake Up.vi"("error in (no error)"=w156, "chanel number (1)"=w158, "DDS ref in"=w157) -> ("error out"=w155:errorcluster)  [unwired: 7 in, 1 out]
            }
          }
        }
      }
      event Value Change {
        n94 = event-data() -> ()  [unwired: 1 in, 5 out]
        n95 = local read "DDS Settings Box 2"() -> (w160:T3)
        n96 = Unbundle By Name(w160) -> ("DDS box device reference"=w163:T5, "DDS Power"=w162:bool[])
        n97 = for {
          N: 4 -> [_]
          tunnel: w163 -> [w168]
          tunnel: w162 -> [w167] mode=indexing
          tunnel: w161 -> [w166]
          tunnel: [w165] -> w159
          i -> [w170]
          n98 = Increment(x=w170) -> (x+1=w169:i32)
          n99 = case shown="True" w167 {
            tunnel: w169 -> [w174 w178]
            tunnel: w168 -> [w173 w177]
            tunnel: w166 -> [w172 w176]
            tunnel: [w171 w175] -> w165
            frame False {
              n100 = call "DDS Power Down.vi"("error in (no error)"=w172, "chanel number (1)"=w174, "DDS ref in"=w173) -> ("error out"=w171:errorcluster)  [unwired: 7 in, 1 out]
            }
            frame True {
              n101 = call "DDS Wake Up.vi"("error in (no error)"=w176, "chanel number (1)"=w178, "DDS ref in"=w177) -> ("error out"=w175:errorcluster)  [unwired: 7 in, 1 out]
            }
          }
        }
      }
      event Value Change {
        n102 = event-data() -> ()  [unwired: 1 in, 5 out]
        n103 = local read "DDS Settings Box 1"() -> (w180:T3)
        n104 = Unbundle By Name(w180) -> ("DDS Profile #"=w179:u8)
        n105 = Build Array(w179, u8 0 ("element"), u8 0 ("element")) -> (w182:u8[])
        n106 = Build Array(u8 0 ("element"), w179) -> (w184:u8[])
        n107 = property on="RAM Function Settings" class="Arr (strict)"("Index Values"=w182) -> ()  [unwired: 2 in, 2 out]
        n108 = property on="RAM Static Array" class="Arr (strict)"("Index Values"=w182) -> ()  [unwired: 2 in, 2 out]
        n109 = property on="DDS Power" class="Arr (strict)"("Index Values"=w184) -> ()  [unwired: 2 in, 2 out]
        n110 = property on="Single Tone Profiles" class="Arr (strict)"("Index Values"=w184) -> ()  [unwired: 2 in, 2 out]
        n111 = property on="RAM Mode" class="Arr (strict)"("Index Values"=w184) -> ()  [unwired: 2 in, 2 out]
        n112 = property on="Function/Static" class="Arr (strict)"("Index Values"=w184) -> ()  [unwired: 2 in, 2 out]
        n113 = property on="Zero-crossing" class="Arr (strict)"("Index Values"=w184) -> ()  [unwired: 2 in, 2 out]
        n114 = property on="No Dwell High" class="Arr (strict)"("Index Values"=w184) -> ()  [unwired: 2 in, 2 out]
      }
      event Value Change {
        n115 = event-data() -> ()  [unwired: 1 in, 5 out]
        n116 = local read "DDS Settings Box 2"() -> (w188:T3)
        n117 = Unbundle By Name(w188) -> ("DDS Profile #"=w190:u8)
        n118 = Build Array(u8 0 ("element"), w190) -> (w187:u8[])
        n119 = property on="DDS Power" class="Arr (strict)"("Index Values"=w187) -> ()  [unwired: 2 in, 2 out]
        n120 = property on="Single Tone Profiles" class="Arr (strict)"("Index Values"=w187) -> ()  [unwired: 2 in, 2 out]
        n121 = property on="RAM Mode" class="Arr (strict)"("Index Values"=w187) -> ()  [unwired: 2 in, 2 out]
        n122 = property on="Function/Static" class="Arr (strict)"("Index Values"=w187) -> ()  [unwired: 2 in, 2 out]
        n123 = property on="RAM Function Settings" class="Arr (strict)"("Index Values"=w187) -> ()  [unwired: 2 in, 2 out]
        n124 = property on="RAM Static Array" class="Arr (strict)"("Index Values"=w187) -> ()  [unwired: 2 in, 2 out]
        n125 = property on="Zero-crossing" class="Arr (strict)"("Index Values"=w187) -> ()  [unwired: 2 in, 2 out]
        n126 = property on="No Dwell High" class="Arr (strict)"("Index Values"=w187) -> ()  [unwired: 2 in, 2 out]
      }
      event "Check DDS Box 1": Value Change {
        n127 = event-data() -> ()  [unwired: 1 in, 5 out]
        n128 = local write "Check DDS Box 1"(FALSE ("Check DDS Box 1")) -> ()
        n129 = local read "DDS Settings Box 1"() -> (w200:T3)
        n130 = Unbundle By Name(w200) -> ("DDS box device reference"=w199:T5)
        n131 = for {
          N: 4 -> [_]
          tunnel: w199 -> [w215]
          tunnel: [w204] -> w196 mode=indexing
          tunnel: [w203] -> w195 mode=indexing
          tunnel: [w202] -> w194 mode=indexing
          shift-right: [w201] -> w193
          shift-left: w198 -> [w214]
          i -> [w213]
          n132 = Increment(x=w213) -> (x+1=w205:i32)
          n133 = call "DDS Read Register.vi"("channel number (1)"=w205, "error in (no error)"=w214, "Register"=AD9910_registers."CFR1", "DDS ref in"=w215) -> ("error out"=w210:errorcluster, "Read data"=w204:u8[], "DDS ref out"=w211:T5)  [unwired: 5 in]
          n134 = call "DDS Read Register.vi"("channel number (1)"=w205, "error in (no error)"=w210, "Register"=AD9910_registers."CFR2", "DDS ref in"=w211) -> ("error out"=w209:errorcluster, "Read data"=w203:u8[], "DDS ref out"=w208:T5)  [unwired: 5 in]
          n135 = call "DDS Read Register.vi"("channel number (1)"=w205, "error in (no error)"=w209, "Register"=AD9910_registers."CFR3", "DDS ref in"=w208) -> ("error out"=w201:errorcluster, "Read data"=w202:u8[])  [unwired: 5 in, 1 out]
        }
        "Box 1 CFR1" <- w196
        "Box 1 CFR2" <- w195
        "Box 1 CFR3" <- w194
      }
      event "Check DDS Box 2": Value Change {
        n136 = event-data() -> ()  [unwired: 1 in, 5 out]
        n137 = local write "Check DDS Box 2"(FALSE ("Check DDS Box 2")) -> ()
        n138 = local read "DDS Settings Box 2"() -> (w219:T3)
        n139 = Unbundle By Name(w219) -> ("DDS box device reference"=w224:T5)
        n140 = for {
          N: 4 -> [_]
          tunnel: w224 -> [w239]
          tunnel: [w228] -> w222 mode=indexing
          tunnel: [w227] -> w221 mode=indexing
          tunnel: [w226] -> w220 mode=indexing
          shift-right: [w225] -> w217
          shift-left: w218 -> [w238]
          i -> [w237]
          n141 = Increment(x=w237) -> (x+1=w229:i32)
          n142 = call "DDS Read Register.vi"("channel number (1)"=w229, "error in (no error)"=w238, "Register"=AD9910_registers."CFR1", "DDS ref in"=w239) -> ("error out"=w234:errorcluster, "Read data"=w228:u8[], "DDS ref out"=w235:T5)  [unwired: 5 in]
          n143 = call "DDS Read Register.vi"("channel number (1)"=w229, "error in (no error)"=w234, "Register"=AD9910_registers."CFR2", "DDS ref in"=w235) -> ("error out"=w233:errorcluster, "Read data"=w227:u8[], "DDS ref out"=w232:T5)  [unwired: 5 in]
          n144 = call "DDS Read Register.vi"("channel number (1)"=w229, "error in (no error)"=w233, "Register"=AD9910_registers."CFR3", "DDS ref in"=w232) -> ("error out"=w225:errorcluster, "Read data"=w226:u8[])  [unwired: 5 in, 1 out]
        }
        "Box 2 CFR1" <- w222
        "Box 2 CFR2" <- w221
        "Box 2 CFR3" <- w220
      }
      event "Variable Actions.Load Variables": Value Change {
        w250 = "\n"  # load in each line
        n145 = event-data() -> ()  [unwired: 1 in, 5 out]
        n146 = call-poly <vilib>:"Read From Spreadsheet File.vi"("delimiter (\\t)"=w250) -> ("all rows"=w249:string[][])  [unwired: 6 in, 4 out]
        n147 = Index Array "Convert false 2D array to 1D"(array=w249, index (row)=0) -> (element=w241:string[])  [unwired: 1 in]
        n148 = Delete From Array "Remove Header"(array=w241, length=1, index=0) -> (array with subset deleted=w240:string[])  [unwired: 1 out]
        n149 = for {
          shift-right: [w260] -> w246
          shift-left: w244 -> [w261]
          tunnel: w240 -> [w262] mode=indexing
          tunnel: [w254] -> w245 mode=indexing
          n150 = Scan From String(format string="%s\t%s\t%f\t%f\t%u\n", input string=w262, error in=w261) -> (error out=w260:errorcluster, output 1=w259:string, output 2=w258:string, output 3=w257:dbl, output 4=w256:dbl, output 5=w255:i32)  [unwired: 6 in, 2 out]
          n151 = Bundle By Name(cluster=T10 {"Description"="", "Name (a,a0...a9)"="", "min"=0.0, "max"=0.0, "# steps"=0} ("Cluster"), "Description"=w259, "Name (a,a0...a9)"=w258, "min"=w257, "max"=w256, "# steps"=w255) -> (w254:T10)
        }
        n152 = property on="Variables" class="Arr (strict)"(error in=w246, "Value"=w245) -> (error out=w247:errorcluster)  [unwired: 1 in, 1 out]
        n153 = property on="Load Variables" class="Bool (strict)"(error in=w247, "Value"=FALSE) -> (error out=w252:errorcluster)  [unwired: 1 in, 1 out]
      }
      event "Variable Actions.Load Paramters": Value Change {
        w274 = "\n"  # load in each line
        n154 = event-data() -> ()  [unwired: 1 in, 5 out]
        n155 = call-poly <vilib>:"Read From Spreadsheet File.vi"("delimiter (\\t)"=w274) -> ("all rows"=w273:string[][])  [unwired: 6 in, 4 out]
        n156 = Index Array "Convert false 2D array to 1D"(array=w273, index (row)=0) -> (element=w265:string[])  [unwired: 1 in]
        n157 = Delete From Array "Remove Header"(array=w265, length=1, index=0) -> (array with subset deleted=w264:string[])  [unwired: 1 out]
        n158 = for {
          shift-right: [w283] -> w269
          shift-left: w271 -> [w284]
          tunnel: w264 -> [w285] mode=indexing
          tunnel: [w278] -> w270 mode=indexing
          n159 = Scan From String(format string="%s\t%s\t%s\t%f\n", input string=w285, error in=w284) -> (error out=w283:errorcluster, output 1=w282:string, output 2=w281:string, output 3=w280:string, output 4=w279:dbl)  [unwired: 5 in, 2 out]
          n160 = Bundle By Name(cluster=T11 {"Description"="", "Name (a,a0...a9)"="", "Equation"="", "Result"=0.0} ("Cluster"), "Description"=w282, "Name (a,a0...a9)"=w281, "Equation"=w280, "Result"=w279) -> (w278:T11)
        }
        n161 = property on="Parameters" class="Arr (strict)"(error in=w269, "Value"=w270) -> (error out=w268:errorcluster)  [unwired: 1 in, 1 out]
        n162 = property on="Load Paramters" class="Bool (strict)"(error in=w268, "Value"=FALSE) -> (error out=w276:errorcluster)  [unwired: 1 in, 1 out]
      }
      event "Variable Actions.Save Variables": Value Change {
        n163 = event-data() -> ()  [unwired: 1 in, 5 out]
        n164 = property on="Variables" class="Arr (strict)"(error in=w290) -> (error out=w288:errorcluster, "Value"=w289:T12)  [unwired: 1 in, 1 out]
        n165 = call "save_variables_table.vi"("error in"=w288, "Variable Settings.Variables"=w289) -> ("error out"=w287:errorcluster)  [unwired: 9 in]
        n166 = property on="Return button to the unclicked position" class="Bool (strict)"(error in=w287, "Value"=FALSE) -> (error out=w291:errorcluster)  [unwired: 1 in, 1 out]
      }
      event "Variable Actions.Save Parameters": Value Change {
        n167 = event-data() -> ()  [unwired: 1 in, 5 out]
        n168 = property on="Parameters" class="Arr (strict)"(error in=w296) -> (error out=w294:errorcluster, "Value"=w295:T13)  [unwired: 1 in, 1 out]
        n169 = call "save_parameters_table.vi"("error in"=w294, "Parameters"=w295) -> ("error out"=w293:errorcluster)  [unwired: 9 in]
        n170 = property on="Save Parameters" class="Bool (strict)"(error in=w293, "Value"=FALSE) -> (error out=w298:errorcluster)  [unwired: 1 in, 1 out]
      }
      event "Variable Actions.Clear Log": Value Change {
        n171 = event-data() -> ()  [unwired: 1 in, 5 out]
        n172 = call "append_to_log.vi"("error in"=w301, "Action"=T7."Clear Log") -> ("error out"=w300:errorcluster)  [unwired: 9 in]
        n173 = property on="Clear Log" class="Bool (strict)"(error in=w300, "Value"=FALSE) -> (error out=w299:errorcluster)  [unwired: 1 in, 1 out]
      }
      event "Variable Actions.Evaluate Parameters": Value Change {
        n174 = event-data() -> ()  [unwired: 1 in, 5 out]
        n175 = property on="Parameters" class="Arr (strict)"(error in=w309) -> (error out=w308:errorcluster, "Value"=w307:T13)  [unwired: 1 in, 1 out]
        n176 = for {
          tunnel: [w320] -> w314 mode=indexing
          tunnel: [w319] -> w313 mode=indexing
          tunnel: w307 -> [w318] mode=indexing
          n177 = Unbundle By Name(w318) -> ("Name (a,a0...a9)"=w320:string, "Equation"=w319:string)
        }
        n178 = call "evaluate_notes.vi"("error in (no error)"=w308, "equations"=w313, "variable names"=w314) -> ("error out"=w305:errorcluster, "parameter values"=w312:dbl[])  [unwired: 7 in]
        n179 = for {
          tunnel: w312 -> [w317] mode=indexing
          tunnel: [w316] -> w306 mode=indexing
          tunnel: w307 -> [w315] mode=indexing
          n180 = Bundle By Name(cluster=w315, "Result"=w317) -> (w316:T11)
        }
        n181 = property on="Parameters" class="Arr (strict)"(error in=w305, "Value"=w306) -> (error out=w304:errorcluster)  [unwired: 1 in, 1 out]
        n182 = property on="Evaluate Parameters" class="Bool (strict)"(error in=w304, "Value"=FALSE) -> (error out=w311:errorcluster)  [unwired: 1 in, 1 out]
      }
      event "Initialize DDS Boxes": Value Change {
        n183 = event-data() -> ()  [unwired: 1 in, 5 out]
        n184 = local read "Variable Settings"() -> (w323:T2)
        n185 = call "get_variable_start_values.vi"("Variable Settings"=w323) -> ("variable/parameter names"=w321:string[], "minimum/current values"=w322:dbl[])  [unwired: 9 in]
        n186 = case shown="True" "Initialize DDS Boxes" {
          tunnel: w325 -> [w327 w334]
          tunnel: [w327 w331] -> w324
          tunnel: w321 -> [_ w330]
          tunnel: w322 -> [_ w329]
          frame False {
          }
          frame True {
            # "DDS Box Initialization"
            n187 = Build Array("DDS Settings Box 1", "DDS Settings Box 2") -> (w336:T3[])
            n188 = for {
              N: "DDS # of Boxes" -> [_]
              tunnel: w336 -> [w341] mode=indexing
              shift-right: [w339] -> w331
              shift-left: w334 -> [w340]
              tunnel: w330 -> [w338]
              tunnel: w329 -> [w337]
              # "DDS Box loop"
              n189 = call "DDS Startup.vi"("error in (no error)"=w340, "Variable Names"=w338, "Variable Values"=w337, "DDS Settings"=w341) -> ("error out"=w339:errorcluster)  [unwired: 6 in, 1 out]
            }
            "DDS Initialized" <- TRUE ("DDS Initialized")
          }
        }
      }
      event "Load DDS Data": Value Change {
        n190 = event-data() -> ()  [unwired: 1 in, 5 out]
        n191 = call "load_xml.vi"("error in"=w346) -> ("error out"=w342:errorcluster, "Array of DDS Boxes"=w345:T3[], "DDS # of Boxes"=w344:i32)  [unwired: 7 in, 1 out]
        n192 = property on="DDS # of Boxes" class="DigNum (strict)"(error in=w342, "Value"=w344) -> (error out=w343:errorcluster)  [unwired: 1 in, 1 out]
        n193 = Index Array(array=w345, index=1) -> (element=w347:T3)
        n194 = Index Array(array=w345, index=0) -> (element=w348:T3)
        n195 = local write "DDS Settings Box 2"(w347) -> ()
        n196 = local write "DDS Settings Box 1"(w348) -> ()
      }
      event "Save DDS Data": Value Change {
        n197 = event-data() -> ()  [unwired: 1 in, 5 out]
        n198 = local read "DDS Settings Box 1"() -> (w357:T3)
        n199 = local read "DDS Settings Box 2"() -> (w356:T3)
        n200 = local read "DDS # of Boxes"() -> (w355:i32)
        n201 = Build Array(w357, w356) -> (w354:T3[])
        n202 = call "save_xml.vi"("error in"=w353, "Array of DDS Boxes"=w354, "DDS # of Boxes"=w355, "Enable DDS"=TRUE) -> ("error out"=w352:errorcluster)  [unwired: 7 in]
      }
      event "Quit Program": Value Change {
        n203 = event-data() -> ()  [unwired: 1 in, 5 out]
      }
    }
    n204 = call "handle_errors.vi"("error in (no error)"=w20) -> ("error out"=w18:errorcluster, "Stop"=w17:bool)  [unwired: 9 in]
    n205 = Or(x=w19, y=w17) -> (x .or. y?=w21:bool)
  }
  n206 = local read "DDS Settings Box 1"() -> (w2:T3)
  n207 = local read "DDS Settings Box 2"() -> (w3:T3)
  n208 = Unbundle By Name(w2) -> ("DDS box device reference"=w4:T5)
  n209 = Unbundle By Name(w3) -> ("DDS box device reference"=w5:T5)
  n210 = Build Array(w4, w5) -> (w6:T5[])
  n211 = local read "DDS # of Boxes"() -> (w7:i32)
  n212 = for {
    N: w7 -> [_]
    tunnel: w15 -> [w362]
    tunnel: [w361] -> w8
    tunnel: w6 -> [w360] mode=indexing
    n213 = call "DDS Close.vi"("error in (no error)"=w362, "DDS ref in"=w360) -> ("error out"=w361:errorcluster)  [unwired: 9 in]
  }
  n214 = call <vilib>:"Simple Error Handler.vi"("type of dialog (OK msg:1)"=w16, "error in (no error)"=w8) -> ()  [unwired: 3 in, 5 out]
